vi "Meas Config Panel.vi"(8 "error in":errorcluster, 9 "force no GUI (False)":bool, 10 "always show setup (False)":bool, 11 "session in":T91={"adc"={"niScope"={"channel cfg"=[], "sessions"=[], "multi cards"=FALSE, "channels"=0, "type"=enum."n/a", "memory [B/chn]"=0, "ext. clock [Hz]"=0.0, "samples count"=0, "use streaming"=FALSE, "proc setup"={"packet size [smpl]"=0, "current timeout [s]"=0.0, "blk2blk timeout [s]"=0.0, "event time"=timestamp(0 s since 1904-01-01), "temp sampl T [s]"=0.0, "data queue"=refnum, "stop notifier"=refnum, "proc ref"=refnum}, "sample width [B]"=0, "ranges [V]"=[], "trigger setup"={"coupling"=1, "level [V]"=0.0, "slope"=0, "mode"=enum."Immediate", "pre-trigger [%]"=0.0}, "fs [Hz]"=0.0, "bitres [bit]"=0, "clock source"=enum."VAL_NO_SOURCE"}, "3458A"={"channels"=[], "sync unit"={"VISA"="", "type"=enum."Picotest U6200A"}, "awg unit"={"type"=enum."Agilent 331xxA to 332xxA", "VISA"="", "enable 10MHz ref"=FALSE, "cmi ckd2"={"VISA"="", "clock source"=enum."Auto", "manual ref clk"=FALSE, "ref clock [Hz]"=0.0, "div mode"=enum."Set divisor directly"}, "cmi sync v3"={"VISA"="", "baud rate [bd/s]"=115200, "source"=enum."Auto", "hv range"=enum."1kV", "fsrc is fixed"=FALSE, "fsrc [Hz]"=10000000.0, "freq integ [s]"=1.0, "freq filter"=5, "trig level"=enum."TTL 5V", "chn1 mode"=enum."Source divider", "chn1 level"=enum."Positive 5V", "chn2 mode"=enum."Source divider", "chn2 level"=enum."Positive 5V", "chn2 div"=1, "chn3 mode"=enum."Chn 1 Active", "chn3 level"=enum."Positive 5V", "chn1 div entry"=enum."Calculate nearest divisor from measured fx", "chn1 dev limit [%]"=1.0, "chn1 check dev"=FALSE}, "trigger"={"source"=enum."Immediate", "slope"=enum."POS", "coupling"=enum."DC", "level [V]"=0.0, "hysteresis [V]"=0.0, "pre-trigger [%]"=0.0}, "HMF2500 cfg"={"Baud Rate"=9600, "Parity"=0, "Data Bits"=8, "Flow Control"=4}}, "sync mode"=enum."MASTER-SLAVE, MASTER clocked by TIMER", "streaming mode"=FALSE, "idn mode"=enum."Auto", "sampling mode"=enum."DCV", "sample memory [B]"=0, "proc setup"={"channel id"=0, "packet size [smpl]"=0, "current timeout [s]"=0.0, "blk2blk timeout [s]"=0.0, "event time"=timestamp(0 s since 1904-01-01), "stop notifier"=refnum, "data queues"=[], "proc refs"=[], "bus semaphore"=refnum}, "sample size [B]"=0, "sample count"=0, "aux data"={"channel id"=0, "valid?"=[], "gain [V]"=[], "timestamp [s]"=[], "Ts [s]"=0.0, "abs timestamp"=timestamp(0 s since 1904-01-01), "t [deg C]"=[], "multiplex timestamp [s]"=-1.0, "only multiplex?"=FALSE, "multiplex smpl offset"=0, "overflow?"=FALSE}, "ranges [V]"=[], "aperture [s]"=0.0, "LEVEL trigger"={"edge"=enum."POS", "level [V]"=0.0, "coupling"=enum."DC"}, "trigger mode"=enum."AUTO", "measure temp.?"=FALSE, "disp mesages"=[], "shared bus?"=FALSE, "disable display?"=FALSE, "aper mode"=enum."Manual", "aper rules"=[], "multiplex"={"cycles"=0, "delay [s]"=0.0, "enabled"=FALSE, "overhead [s]"=1.0, "tot smpls"=0, "sub-rec"=0, "overhead [%]"=0.0, "emulated"=FALSE}, "F8588 lpf"=enum."Off", "F8588 pll"=enum."Off", "F8588 couple"=enum."DC, auto", "fs"={"freq mode"=enum."fs or Ts", "fs [Hz]"=0.0, "fref [Hz]"=0.0, "mul"=0.0, "div"=0.0}, "fs mode"=enum."fs or Ts", "init timestamp"=timestamp(0 s since 1904-01-01), "last report timestamp"=timestamp(0 s since 1904-01-01)}, "dsdll"={"dsdll"={"dsdll path"=path "", "dsdll handle"=[], "output devices"=[], "capture devices"=[]}, "channels"=0, "device id"=0, "channel idns"=[], "proc setup"={"packet size [smpl]"=0, "current timeout [s]"=0.0, "blk2blk timeout [s]"=0.0, "event time"=timestamp(0 s since 1904-01-01), "data queue"=refnum, "stop notifier"=refnum, "proc ref"=refnum}, "samples count"=0, "fs [Hz]"=0.0}, "type"=enum."niScope", "channel idn str"=[], "aux instr idn str"=[], "modified?"=FALSE, "simadc"={"channels"=[], "range [V]"=0.0, "Ts step [s]"=0.0, "time [s]"=0.0, "fs [Hz]"=0.0, "count"=0, "smpl offset"=0, "set count"=0, "bit res"=0}, "force rst?"=FALSE, "exit mode"=enum."Immediate reset", "exit dly"=0.0, "exit tmr"=timestamp(0 s since 1904-01-01), "busy?"=FALSE, "accessed?"=FALSE, "multiplex"={"Type"=enum."Dummy", "gen com ssn"={"visa"="", "primary"=enum."None", "secondary"=enum."None", "channels"=[]}, "delay before [s]"=0.0, "delay post [s]"=0.0, "sequence"=[], "enabled"=FALSE, "ref timestamp [s]"=0.0, "idn string"="", "dev niScope"="", "niScope idx"=0, "QPMX ssn"={"visa"="", "switch mode"=enum."Switched by TWM", "sequence"=[], "timing delays"=[], "polarity"=enum."Positive", "ss delay (s)"=2.0, "internal timer (s)"=1.0, "Last loaded sequence file"=path "", "startup delay (s)"=2.0}, "VISA mux ssn"={"VISA"="", "paths"=[], "idn command"="", "serial cfg"={"Baud rate"=9600, "Data bits"=8, "Parity"=0, "Stop bits"=10, "Flow control"=0, "End Mode Read"=enum."None", "End Mode Write"=enum."None", "Term character"=0, "Term enable"=FALSE}}}, "keysight dso"={"VISA"="", "channels"=[], "bw limit [Hz]"=0.0, "resolution"=enum."Basic", "trig noise reject"=enum."Normal", "N"=0, "trigger config"={"trigger source"=enum."Immediate", "trigger slope"=enum."Negative", "level [V]"=0.0, "hysteresis [V]"=0.001, "pre-trig [%]"=50}, "fs [Hz]"=0.0, "timeout stop"=timestamp(0 s since 1904-01-01), "waiting for opc"=FALSE, "fetch offset [smpl]"=0, "abs timestamp"=timestamp(0 s since 1904-01-01), "ranges [V]"=[], "decimation"=1.0, "ext ref"=FALSE, "emulate aperture"=FALSE, "model"=enum."DSO91304"}, "cdaq"={"mclk [Hz]"=12800000.0, "ADC task"="", "mclk reference"="", "fs [Hz]"=50000.0, "queue adc cmd"=refnum, "queue adc data"=refnum, "adc proc ref"=refnum, "channels"=[], "last channels"=[], "timeout"=timestamp(0 s since 1904-01-01), "N"=1000, "mclk mode"=enum."Free running", "ext mclk source"=""}, "ignore overload"=FALSE, "ADS127L21"={"VISA"="", "chn list"=[], "record size"=0, "phys. channels"=0, "adc fifo size"=0, "channels"=[], "ext refclk?"=FALSE, "fs [Hz]"=0.0, "ext refclk [Hz]"=0.0, "meas refclk [Hz]"=0.0, "EXTOUT mode"=enum."ADCCLK", "EXTOUT polarity"=enum."NORM", "EXTOUT divisor"=0}}, "sequence"=[], "sequence setup"={"group setups"=[], "rec count"=0, "range mode"=enum."Keep defaults", "fs mode"=enum."Frequency", "rng even"=0.0, "rng odd"=0.0, "folder"=path "", "name base"="", "meas id"=0, "settle [s]"=0.0, "comment"="", "avg count"=0, "fs-abs-fr fr"=0.0, "fs-abs-fr fs"=0.0, "fs-div fr"=0.0, "fs-div div"=0.0, "fs-mn fr"=0.0, "fs-mn mul"=0.0, "fs-mn div"=0.0, "fs-rat fr"=0.0, "fs-rat rat"=0.0}, "golpi"=refnum, "processing setup"={"mode"=enum."Raw", "call after avgs?"=FALSE, "calculate?"=FALSE, "raw mode"={"command"="", "result mode"=enum."Display console output (only Octave)", "res variable"=""}, "QWTB"={"QWTB path"=path "", "alg filter path"="", "alg ids"=[], "alg parameters"=[], "parsed parameters"=[], "selected alg id"="", "selected unc mode"=enum."None", "qwtb mcc"=100, "qwtb timeout"=90, "qwtb covg"=95.0, "qwtb ofs"=0, "qwtb lim data"=0, "multicore"={"jobs folder"=path "", "cores"=0, "max jobs"=0, "mode"=enum."Singlecore"}, "unc once?"=FALSE, "qwtb tstemp"=enum."Enabled (default)", "octave reset"=FALSE, "exec mode"=enum."Single-core"}}, "corrections"={"transducers"={"channels"=[], "last path"=path "", "root path"=path ""}, "digitizer"={"last path"=path "", "channel paths"=[], "channel idns"=[], "correction name"="", "channel names"=[], "folders to copy"=[], "channel valid"=[], "correction path"=path "", "correction rel path"="", "rel folders to copy"=[], "root path"=path ""}}, "assist cfg"={"P"=0, "Q"=0, "rel shift"=0.0, "ref freq"=0.0, "min fs"=0.0, "max fs tol"=0.0, "min int"=0.0, "max int"=0.0, "max err"=0.0, "max timeout"=0.0}} {"corrections"."transducers"."channels"."Phase index" min=1 step=1; "adc"."ADS127L21"."channels"."Channel" min=1 max=8 step=1; "adc"."ADS127L21"."channels"."Range [Vpk]" items=["±1.65V", "±2V"]; "adc"."cdaq"."last channels"."Channel id" min=0 step=1; "adc"."cdaq"."channels"."Channel id" min=0 step=1; "adc"."keysight dso"."decimation" min=1.0; "adc"."keysight dso"."bw limit [Hz]" format="%#_6p"; "adc"."keysight dso"."channels"."Offset [V]" format="%#_6p"; "adc"."keysight dso"."channels"."Range [Vpk]" min=0.0 format="%#_6p"; "adc"."keysight dso"."channels"."Channel" min=1; "adc"."multiplex"."VISA mux ssn"."serial cfg"."Flow control" items=["None", "XON/XOFF", "CTS/RTS", "XON/XOFF + CTS/RTS", "DTR/DSR", "XON/XOFF + DTR/DSR"]; "adc"."multiplex"."VISA mux ssn"."serial cfg"."Stop bits" items=["1 bit"=10, "1.5 bits"=15, "2 bits"=20]; "adc"."multiplex"."VISA mux ssn"."serial cfg"."Parity" items=["None", "Odd", "Even", "Mark", "Space"]; "adc"."multiplex"."VISA mux ssn"."serial cfg"."Data bits" items=["5 bits"=5, "6 bits"=6, "7 bits"=7, "8 bits"=8]; "adc"."multiplex"."VISA mux ssn"."serial cfg"."Baud rate" items=["150 Bd"=150, "300 Bd"=300, "600 Bd"=600, "1200 Bd"=1200, "2400 Bd"=2400, "4800 Bd"=4800, "9600 Bd"=9600, "19.2 kBd"=19200, "38.4 kBd"=38400, "57.6 kBd"=57600, "115.2 kBd"=115200]; "adc"."multiplex"."QPMX ssn"."startup delay (s)" min=0.0 step=1.0; "adc"."multiplex"."QPMX ssn"."internal timer (s)" min=0.0 step=1.0; "adc"."multiplex"."QPMX ssn"."ss delay (s)" min=0.0 step=1.0; "adc"."multiplex"."QPMX ssn"."timing delays" min=1 max=255 step=1; "adc"."3458A"."awg unit"."HMF2500 cfg"."Flow Control" items=["None", "XON/XOFF", "RTS/CTS", "XON/XOFF & RTS/CTS", "DTR/DSR", "XON/XOFF & DTR/DSR"]; "adc"."3458A"."awg unit"."HMF2500 cfg"."Data Bits" items=["7"=7, "8"=8]; "adc"."3458A"."awg unit"."HMF2500 cfg"."Parity" items=["None", "Odd", "Even", "Mark", "Space"]; "adc"."3458A"."awg unit"."HMF2500 cfg"."Baud Rate" items=["300"=300, "600"=600, "1200"=1200, "2400"=2400, "4800"=4800, "9600"=9600, "19200"=19200]; "adc"."3458A"."awg unit"."cmi sync v3"."chn2 div" min=1 max=100000000 step=1; "adc"."3458A"."awg unit"."cmi sync v3"."fsrc [Hz]" format="%_8p"; "adc"."3458A"."channels"."Range [Vpk]" min=0.0; "adc"."niScope"."trigger setup"."pre-trigger [%]" format="%.2f"; "adc"."niScope"."trigger setup"."level [V]" format="%.2f"; "adc"."niScope"."trigger setup"."coupling" items=["AC"=0, "DC"=1, "HF Reject"=3, "LF Reject"=4, "AC Plus HF Reject"=1001]; "adc"."niScope"."channel cfg"."Range [Vpk]" min=0.0; "adc"."niScope"."channel cfg"."Channel" min=0}) -> (0 "error out":errorcluster, 2 "canceled?":bool, 3 "session out":T91={"adc"={"niScope"={"channel cfg"=[], "sessions"=[], "multi cards"=FALSE, "channels"=0, "type"=enum."n/a", "memory [B/chn]"=0, "ext. clock [Hz]"=0.0, "samples count"=0, "use streaming"=FALSE, "proc setup"={"packet size [smpl]"=0, "current timeout [s]"=0.0, "blk2blk timeout [s]"=0.0, "event time"=timestamp(0 s since 1904-01-01), "temp sampl T [s]"=0.0, "data queue"=refnum, "stop notifier"=refnum, "proc ref"=refnum}, "sample width [B]"=0, "ranges [V]"=[], "trigger setup"={"coupling"=1, "level [V]"=0.0, "slope"=0, "mode"=enum."Immediate", "pre-trigger [%]"=0.0}, "fs [Hz]"=0.0, "bitres [bit]"=0, "clock source"=enum."VAL_NO_SOURCE"}, "3458A"={"channels"=[], "sync unit"={"VISA"="", "type"=enum."Picotest U6200A"}, "awg unit"={"type"=enum."Agilent 331xxA to 332xxA", "VISA"="", "enable 10MHz ref"=FALSE, "cmi ckd2"={"VISA"="", "clock source"=enum."Auto", "manual ref clk"=FALSE, "ref clock [Hz]"=0.0, "div mode"=enum."Set divisor directly"}, "cmi sync v3"={"VISA"="", "baud rate [bd/s]"=115200, "source"=enum."Auto", "hv range"=enum."1kV", "fsrc is fixed"=FALSE, "fsrc [Hz]"=10000000.0, "freq integ [s]"=1.0, "freq filter"=5, "trig level"=enum."TTL 5V", "chn1 mode"=enum."Source divider", "chn1 level"=enum."Positive 5V", "chn2 mode"=enum."Source divider", "chn2 level"=enum."Positive 5V", "chn2 div"=1, "chn3 mode"=enum."Chn 1 Active", "chn3 level"=enum."Positive 5V", "chn1 div entry"=enum."Calculate nearest divisor from measured fx", "chn1 dev limit [%]"=1.0, "chn1 check dev"=FALSE}, "trigger"={"source"=enum."Immediate", "slope"=enum."POS", "coupling"=enum."DC", "level [V]"=0.0, "hysteresis [V]"=0.0, "pre-trigger [%]"=0.0}, "HMF2500 cfg"={"Baud Rate"=9600, "Parity"=0, "Data Bits"=8, "Flow Control"=4}}, "sync mode"=enum."MASTER-SLAVE, MASTER clocked by TIMER", "streaming mode"=FALSE, "idn mode"=enum."Auto", "sampling mode"=enum."DCV", "sample memory [B]"=0, "proc setup"={"channel id"=0, "packet size [smpl]"=0, "current timeout [s]"=0.0, "blk2blk timeout [s]"=0.0, "event time"=timestamp(0 s since 1904-01-01), "stop notifier"=refnum, "data queues"=[], "proc refs"=[], "bus semaphore"=refnum}, "sample size [B]"=0, "sample count"=0, "aux data"={"channel id"=0, "valid?"=[], "gain [V]"=[], "timestamp [s]"=[], "Ts [s]"=0.0, "abs timestamp"=timestamp(0 s since 1904-01-01), "t [deg C]"=[], "multiplex timestamp [s]"=-1.0, "only multiplex?"=FALSE, "multiplex smpl offset"=0, "overflow?"=FALSE}, "ranges [V]"=[], "aperture [s]"=0.0, "LEVEL trigger"={"edge"=enum."POS", "level [V]"=0.0, "coupling"=enum."DC"}, "trigger mode"=enum."AUTO", "measure temp.?"=FALSE, "disp mesages"=[], "shared bus?"=FALSE, "disable display?"=FALSE, "aper mode"=enum."Manual", "aper rules"=[], "multiplex"={"cycles"=0, "delay [s]"=0.0, "enabled"=FALSE, "overhead [s]"=1.0, "tot smpls"=0, "sub-rec"=0, "overhead [%]"=0.0, "emulated"=FALSE}, "F8588 lpf"=enum."Off", "F8588 pll"=enum."Off", "F8588 couple"=enum."DC, auto", "fs"={"freq mode"=enum."fs or Ts", "fs [Hz]"=0.0, "fref [Hz]"=0.0, "mul"=0.0, "div"=0.0}, "fs mode"=enum."fs or Ts", "init timestamp"=timestamp(0 s since 1904-01-01), "last report timestamp"=timestamp(0 s since 1904-01-01)}, "dsdll"={"dsdll"={"dsdll path"=path "", "dsdll handle"=[], "output devices"=[], "capture devices"=[]}, "channels"=0, "device id"=0, "channel idns"=[], "proc setup"={"packet size [smpl]"=0, "current timeout [s]"=0.0, "blk2blk timeout [s]"=0.0, "event time"=timestamp(0 s since 1904-01-01), "data queue"=refnum, "stop notifier"=refnum, "proc ref"=refnum}, "samples count"=0, "fs [Hz]"=0.0}, "type"=enum."niScope", "channel idn str"=[], "aux instr idn str"=[], "modified?"=FALSE, "simadc"={"channels"=[], "range [V]"=0.0, "Ts step [s]"=0.0, "time [s]"=0.0, "fs [Hz]"=0.0, "count"=0, "smpl offset"=0, "set count"=0, "bit res"=0}, "force rst?"=FALSE, "exit mode"=enum."Immediate reset", "exit dly"=0.0, "exit tmr"=timestamp(0 s since 1904-01-01), "busy?"=FALSE, "accessed?"=FALSE, "multiplex"={"Type"=enum."Dummy", "gen com ssn"={"visa"="", "primary"=enum."None", "secondary"=enum."None", "channels"=[]}, "delay before [s]"=0.0, "delay post [s]"=0.0, "sequence"=[], "enabled"=FALSE, "ref timestamp [s]"=0.0, "idn string"="", "dev niScope"="", "niScope idx"=0, "QPMX ssn"={"visa"="", "switch mode"=enum."Switched by TWM", "sequence"=[], "timing delays"=[], "polarity"=enum."Positive", "ss delay (s)"=2.0, "internal timer (s)"=1.0, "Last loaded sequence file"=path "", "startup delay (s)"=2.0}, "VISA mux ssn"={"VISA"="", "paths"=[], "idn command"="", "serial cfg"={"Baud rate"=9600, "Data bits"=8, "Parity"=0, "Stop bits"=10, "Flow control"=0, "End Mode Read"=enum."None", "End Mode Write"=enum."None", "Term character"=0, "Term enable"=FALSE}}}, "keysight dso"={"VISA"="", "channels"=[], "bw limit [Hz]"=0.0, "resolution"=enum."Basic", "trig noise reject"=enum."Normal", "N"=0, "trigger config"={"trigger source"=enum."Immediate", "trigger slope"=enum."Negative", "level [V]"=0.0, "hysteresis [V]"=0.001, "pre-trig [%]"=50}, "fs [Hz]"=0.0, "timeout stop"=timestamp(0 s since 1904-01-01), "waiting for opc"=FALSE, "fetch offset [smpl]"=0, "abs timestamp"=timestamp(0 s since 1904-01-01), "ranges [V]"=[], "decimation"=1.0, "ext ref"=FALSE, "emulate aperture"=FALSE, "model"=enum."DSO91304"}, "cdaq"={"mclk [Hz]"=12800000.0, "ADC task"="", "mclk reference"="", "fs [Hz]"=50000.0, "queue adc cmd"=refnum, "queue adc data"=refnum, "adc proc ref"=refnum, "channels"=[], "last channels"=[], "timeout"=timestamp(0 s since 1904-01-01), "N"=1000, "mclk mode"=enum."Free running", "ext mclk source"=""}, "ignore overload"=FALSE, "ADS127L21"={"VISA"="", "chn list"=[], "record size"=0, "phys. channels"=0, "adc fifo size"=0, "channels"=[], "ext refclk?"=FALSE, "fs [Hz]"=0.0, "ext refclk [Hz]"=0.0, "meas refclk [Hz]"=0.0, "EXTOUT mode"=enum."ADCCLK", "EXTOUT polarity"=enum."NORM", "EXTOUT divisor"=0}}, "sequence"=[], "sequence setup"={"group setups"=[], "rec count"=0, "range mode"=enum."Keep defaults", "fs mode"=enum."Frequency", "rng even"=0.0, "rng odd"=0.0, "folder"=path "", "name base"="", "meas id"=0, "settle [s]"=0.0, "comment"="", "avg count"=0, "fs-abs-fr fr"=0.0, "fs-abs-fr fs"=0.0, "fs-div fr"=0.0, "fs-div div"=0.0, "fs-mn fr"=0.0, "fs-mn mul"=0.0, "fs-mn div"=0.0, "fs-rat fr"=0.0, "fs-rat rat"=0.0}, "golpi"=refnum, "processing setup"={"mode"=enum."Raw", "call after avgs?"=FALSE, "calculate?"=FALSE, "raw mode"={"command"="", "result mode"=enum."Display console output (only Octave)", "res variable"=""}, "QWTB"={"QWTB path"=path "", "alg filter path"="", "alg ids"=[], "alg parameters"=[], "parsed parameters"=[], "selected alg id"="", "selected unc mode"=enum."None", "qwtb mcc"=100, "qwtb timeout"=90, "qwtb covg"=95.0, "qwtb ofs"=0, "qwtb lim data"=0, "multicore"={"jobs folder"=path "", "cores"=0, "max jobs"=0, "mode"=enum."Singlecore"}, "unc once?"=FALSE, "qwtb tstemp"=enum."Enabled (default)", "octave reset"=FALSE, "exec mode"=enum."Single-core"}}, "corrections"={"transducers"={"channels"=[], "last path"=path "", "root path"=path ""}, "digitizer"={"last path"=path "", "channel paths"=[], "channel idns"=[], "correction name"="", "channel names"=[], "folders to copy"=[], "channel valid"=[], "correction path"=path "", "correction rel path"="", "rel folders to copy"=[], "root path"=path ""}}, "assist cfg"={"P"=0, "Q"=0, "rel shift"=0.0, "ref freq"=0.0, "min fs"=0.0, "max fs tol"=0.0, "min int"=0.0, "max int"=0.0, "max err"=0.0, "max timeout"=0.0}} {"corrections"."transducers"."channels"."Phase index" min=1 step=1; "adc"."ADS127L21"."channels"."Channel" min=1 max=8 step=1; "adc"."ADS127L21"."channels"."Range [Vpk]" items=["±1.65V", "±2V"]; "adc"."cdaq"."last channels"."Channel id" min=0 step=1; "adc"."cdaq"."channels"."Channel id" min=0 step=1; "adc"."keysight dso"."decimation" min=1.0; "adc"."keysight dso"."bw limit [Hz]" format="%#_6p"; "adc"."keysight dso"."channels"."Offset [V]" format="%#_6p"; "adc"."keysight dso"."channels"."Range [Vpk]" min=0.0 format="%#_6p"; "adc"."keysight dso"."channels"."Channel" min=1; "adc"."multiplex"."VISA mux ssn"."serial cfg"."Flow control" items=["None", "XON/XOFF", "CTS/RTS", "XON/XOFF + CTS/RTS", "DTR/DSR", "XON/XOFF + DTR/DSR"]; "adc"."multiplex"."VISA mux ssn"."serial cfg"."Stop bits" items=["1 bit"=10, "1.5 bits"=15, "2 bits"=20]; "adc"."multiplex"."VISA mux ssn"."serial cfg"."Parity" items=["None", "Odd", "Even", "Mark", "Space"]; "adc"."multiplex"."VISA mux ssn"."serial cfg"."Data bits" items=["5 bits"=5, "6 bits"=6, "7 bits"=7, "8 bits"=8]; "adc"."multiplex"."VISA mux ssn"."serial cfg"."Baud rate" items=["150 Bd"=150, "300 Bd"=300, "600 Bd"=600, "1200 Bd"=1200, "2400 Bd"=2400, "4800 Bd"=4800, "9600 Bd"=9600, "19.2 kBd"=19200, "38.4 kBd"=38400, "57.6 kBd"=57600, "115.2 kBd"=115200]; "adc"."multiplex"."QPMX ssn"."startup delay (s)" min=0.0 step=1.0; "adc"."multiplex"."QPMX ssn"."internal timer (s)" min=0.0 step=1.0; "adc"."multiplex"."QPMX ssn"."ss delay (s)" min=0.0 step=1.0; "adc"."multiplex"."QPMX ssn"."timing delays" min=1 max=255 step=1; "adc"."3458A"."awg unit"."HMF2500 cfg"."Flow Control" items=["None", "XON/XOFF", "RTS/CTS", "XON/XOFF & RTS/CTS", "DTR/DSR", "XON/XOFF & DTR/DSR"]; "adc"."3458A"."awg unit"."HMF2500 cfg"."Data Bits" items=["7"=7, "8"=8]; "adc"."3458A"."awg unit"."HMF2500 cfg"."Parity" items=["None", "Odd", "Even", "Mark", "Space"]; "adc"."3458A"."awg unit"."HMF2500 cfg"."Baud Rate" items=["300"=300, "600"=600, "1200"=1200, "2400"=2400, "4800"=4800, "9600"=9600, "19200"=19200]; "adc"."3458A"."awg unit"."cmi sync v3"."chn2 div" min=1 max=100000000 step=1; "adc"."3458A"."awg unit"."cmi sync v3"."fsrc [Hz]" format="%_8p"; "adc"."3458A"."channels"."Range [Vpk]" min=0.0; "adc"."niScope"."trigger setup"."pre-trigger [%]" format="%.2f"; "adc"."niScope"."trigger setup"."level [V]" format="%.2f"; "adc"."niScope"."trigger setup"."coupling" items=["AC"=0, "DC"=1, "HF Reject"=3, "LF Reject"=4, "AC Plus HF Reject"=1001]; "adc"."niScope"."channel cfg"."Range [Vpk]" min=0.0; "adc"."niScope"."channel cfg"."Channel" min=0})   [LabVIEW 2020]
doc: "New measurement configuration panel."
uses:
  Meas Session.ctl
  adc/ADC Session.ctl
  drivers/niScope/niScope Session.ctl
  drivers/niScope/niScope Virtual Channel Config.ctl
  drivers/niScope/niScope Virtual Channel Mode.ctl
  drivers/niScope/niScope Virtual Channel Input Z.ctl
  drivers/niScope/niScope Virtual Channel Coupling.ctl
  drivers/niScope/niScope Type.ctl
  drivers/niScope/niScope Digitizing Process Options.ctl
  drivers/niScope/niScope Data Packet.ctl
  drivers/niScope/niScope Trigger Setup.ctl
  <instrlib>/niScope/Controls/niScope trigger coupling.ctl
  <instrlib>/niScope/Controls/niScope trigger slope.ctl
  drivers/niScope/niScope Reference Clock.ctl
  drivers/DMM/3458A Digitizer Session.ctl
  drivers/DMM/3458A Virtual Channel Config.ctl
  drivers/Counter/Counter Session.ctl
  drivers/Counter/Counter Type.ctl
  drivers/AWG/AWG Session.ctl
  drivers/AWG/AWG Type.ctl
  drivers/AWG/CMI Clock Divider v2/CMI ckd2 Session.ctl
  drivers/AWG/CMI Clock Divider v2/CMI ckd2 Source Mode.ctl
  drivers/AWG/CMI Clock Divider v2/CMI ckd2 Divisor Mode.ctl
  drivers/AWG/CMI Sync V3/CMI Sync V3 session.ctl
  drivers/AWG/CMI Sync V3/Configure/CMI Sync V3 Reference Clock Source.ctl
  drivers/AWG/CMI Sync V3/Configure/CMI Sync V3 HV input Range.ctl
  drivers/AWG/CMI Sync V3/Configure/CMI Sync V3 Trigger Input Level.ctl
  drivers/AWG/CMI Sync V3/Configure/CMI Sync V3 Channel 1 Mode.ctl
  drivers/AWG/CMI Sync V3/Configure/CMI Sync V3 Channel Output Levels.ctl
  drivers/AWG/CMI Sync V3/Configure/CMI Sync V3 Channel 2 Mode.ctl
  drivers/AWG/CMI Sync V3/Configure/CMI Sync V3 Channel 3 Mode.ctl
  drivers/AWG/CMI Sync V3/Configure/CMI Sync V3 Channel 1 Divisor Entry Mode.ctl
  adc/ADC Trig Config.ctl
  adc/ADC Trig Mode Source.ctl
  adc/ADC Trig Slope.ctl
  adc/ADC Trig Coupling.ctl
  drivers/AWG/RaS HMF2500/HMF2500 Config.ctl
  drivers/DMM/3458A Sync Mode.ctl
  drivers/DMM/3458A Idn Mode.ctl
  drivers/DMM/3458A Digitizing Low Levels/Configure/Sampling Mode.ctl
  drivers/DMM/3458A Digitizing Process Options.ctl
  drivers/DMM/3458A Data Packet.ctl
  drivers/DMM/3458A Aux Record Data.ctl
  drivers/DMM/3458A Digitizing Low Levels/Configure/Level Setup.ctl
  drivers/DMM/3458A Digitizing Low Levels/Configure/First Sample Trigger.ctl
  drivers/DMM/3458A Aperture Selection Mode.ctl
  drivers/DMM/3458A Multiplexing Config.ctl
  drivers/Fluke 8588A/F8588A Low Pass Filter.ctl
  drivers/Fluke 8588A/F8588A Phase Lock.ctl
  drivers/Fluke 8588A/F8588A Coupling.ctl
  drivers/DMM/3458A Sampling Rate.ctl
  drivers/AWG/AWG Clock Setup Mode.ctl
  drivers/DMM/3458A Sample Rate Mode.ctl
  drivers/dsdll/DSDLL Session.ctl
  drivers/dsdll/dsdll/dsdll_instance.ctl
  drivers/dsdll/dsdll/dsdll_device_record.ctl
  drivers/dsdll/DSDLL Process Config.ctl
  drivers/dsdll/DSDLL Data Packet.ctl
  adc/ADC Type.ctl
  drivers/simulated_adc/SimAdc Config.ctl
  drivers/simulated_adc/SimAdc Channel Cfg.ctl
  adc/ADC On Close Action.ctl
  adc/Multiplexer/MPX Session.ctl
  adc/Multiplexer/MPX Type.ctl
  drivers/Multiplexers/Generic COM/GCOMM Session.ctl
  drivers/Multiplexers/Generic COM/GCOMM Signal.ctl
  drivers/Multiplexers/Generic COM/GCOMM Virtual Channel.ctl
  drivers/Multiplexers/Generic COM/GCOMM Logic State.ctl
  drivers/Multiplexers/Generic COM/QPMX Session.ctl
  drivers/Multiplexers/QPMX/QPMX switch mode.ctl
  drivers/Multiplexers/QPMX/QPMX polarity.ctl
  drivers/Multiplexers/Generic VISA commands/GVISA Mux Session.ctl
  drivers/Multiplexers/Generic VISA commands/GVISA Mux Path Entry.ctl
  drivers/Multiplexers/Generic VISA commands/met_serial_setup.ctl
  drivers/Agilent DSO 90000/Virtual Digitizer/KeDSO session.ctl
  drivers/Agilent DSO 90000/Virtual Digitizer/KeDSO Virtual Channel.ctl
  drivers/Agilent DSO 90000/Virtual Digitizer/KeDSO High Resolution Mode.ctl
  drivers/Agilent DSO 90000/Virtual Digitizer/KeDSO Trigger Setup.ctl
  drivers/Agilent DSO 90000/Virtual Digitizer/KeDSO Trigger Source.ctl
  drivers/Agilent DSO 90000/Public/Utility/DSO type.ctl
  drivers/cdaq/cDAQ Session.ctl
  drivers/cdaq/low_level_old/cdaq_anal_adc_command.ctl
  drivers/cdaq/low_level_old/cdaq_anal_adc_data.ctl
  drivers/cdaq/cDAQ Virtual Channel.ctl
  drivers/cdaq/cDAQ Master Clock Mode.ctl
  drivers/CMI_ADS127L21/CMI ADS127L21 - Session.ctl
  drivers/CMI_ADS127L21/CMI ADS127L21 - Record Channel.ctl
  drivers/CMI_ADS127L21/CMI ADS127L21 - Input Range.ctl
  drivers/CMI_ADS127L21/CMI ADS127L21 - Input Mode.ctl
  drivers/CMI_ADS127L21/CMI ADS127L21 - Input Impedance.ctl
  drivers/CMI_ADS127L21/CMI ADS127L21 - EXTOUT Mode.ctl
  drivers/CMI_ADS127L21/CMI ADS127L21 - EXTOUT Polarity.ctl
  Meas Sequence Item.ctl
  Meas Sampling Configuration.ctl
  processing/QWTB/Meas Proc QWTB Algorithm Parameter Data.ctl
  Meas Sequence Configuration.ctl
  Meas Range Mode.ctl
  Meas Sampling Rate Mode.ctl
  octave/golpi/mpc/golpi_session_ref.ctl
  octave/golpi/mpc/golpi_session.ctl
  octave/golpi/GOLPI reference Type Def.ctl
  octave/golpi/Pipe Handle.ctl
  processing/Meas Process Config.ctl
  processing/Meas Process Mode.ctl
  processing/Meas Process Raw Config.ctl
  processing/Meas Process Raw Result Mode.ctl
  processing/QWTB/Meas Proc QWTB Setup.ctl
  processing/QWTB/Meas Proc QWTB Uncertainty Mode.ctl
  processing/QWTB/Meas Proc QWTB Multicore Setup.ctl
  processing/QWTB/Meas Proc QWTB Multicore Type.ctl
  processing/Meas Process Time Stamp Mode.ctl
  processing/QWTB/Meas Proc QWTB Exec Mode.ctl
  Corrections/Corr Setup.ctl
  Corrections/Corr Tranducer Item.ctl
  Corrections/Corr Digitizers.ctl
  Assist/Assist Panel Setup.ctl
  varilib/SGUI Assign References Mode.ctl
  other/GUI Panel Control Action.ctl
  adc/ADC Capabilities Parameters.ctl
  varilib/SGUI Set Multiple Reals By Label.vi
  varilib/SGUI Set Single Real By Label.vi
  varilib/SGUI Set Single Integer By Label.vi
  varilib/varilib.lvlib
  drivers/AWG/AWG.lvlib
  drivers/DMM/3458A Virtual Digitizer.lvlib
  drivers/niScope/niScope Virtual Digitizer.lvlib
  drivers/Counter/Counter.lvlib
  drivers/DMM/3458A Digitizing Low Levels/3458A Digitizing Low Levels.lvlib
  drivers/dsdll/DSDLL Virtual Digitizer.lvlib
  octave/golpi/GOLPI library.lvlib
  octave/golpi/mpc/GOLPI Multi Process.lvlib
  drivers/dsdll/dsdll/dsdll.lvlib
  octave/golpi/LV Process library.lvlib
  drivers/AWG/CMI Sync V3/CMI Sync Unit V3.lvlib
  drivers/Agilent DSO 90000/Agilent 90000 Series.lvlib
panel:
  in  "pre-trig ratio":dbl=1e-06 caption="Pre-trigger ratio [%]" min=0.0 max=100.0 step=1.0 format="%#_3f"
  in  "trig hyst":dbl=1e-06 caption="Hysteresis [V]" min=1e-06 format="%#_3p"
  in  "btn default":bool
  in  "srate tabs":T1(tab)
  in  "fs mode":T2 caption="Sampling rate mode"
  in  "smpl rate":dbl caption="Sampling rate [Hz]" min=0.0 format="%_9p"
  out "smpl rate min":dbl caption="Sampling rate range [Hz]" format="%#_5p"
  out "smpl rate max":dbl caption="smpl rate min" format="%#_5p"
  out "smpl rate abs fr min":dbl caption="Sampling rate range [Hz]" format="%#_5p"
  out "smpl rate abs fr max":dbl caption="smpl rate min" format="%#_5p"
  in  "smpl abs fr fs":dbl caption="Sampling rate [Hz]" min=0.0 format="%_8p"
  in  "smpl abs fr":dbl caption="Reference frequency [Hz]" min=0.0 format="%_8p"
  out "smpl rate fr/N min":dbl caption="Sampling rate range [Hz]" format="%#_5p"
  out "smpl rate fr/N max":dbl caption="smpl rate min" format="%#_5p"
  out "smpl fr/N fs":dbl caption="Sampling rate [Hz]" min=0.0 format="%_8p"
  in  "smpl fr/N div":dbl=1.0 caption="Divisor" min=1.0 max=10000000.0 step=1.0
  in  "smpl fr/N fr":dbl caption="Reference frequency [Hz]" min=0.0 format="%_8p"
  in  "smpl fr*M/N mul":dbl=1.0 caption="Multiplier" min=1.0 max=10000000.0 step=1.0
  out "smpl rate fr*M/N min":dbl caption="Sampling rate range [Hz]" format="%#_5p"
  out "smpl rate fr*M/N max":dbl caption="smpl rate min" format="%#_5p"
  out "smpl fr*M/N fs":dbl caption="Sampling rate [Hz]" min=0.0 format="%_8p"
  in  "smpl fr*M/N div":dbl=1.0 caption="Divisor" min=1.0 max=10000000.0 step=1.0
  in  "smpl fr*M/N fr":dbl caption="Reference freq [Hz]" min=0.0 format="%_8p"
  in  "smpl fr*R fr":dbl caption="Reference frequency [Hz]" min=0.0 format="%_8p"
  in  "smpl fr*R rat":dbl=1.0 caption="Ratio" min=0.0 max=100000000.0 step=0.1 format="%_8g"
  out "smpl fr*R fs":dbl caption="Sampling rate [Hz]" min=0.0 format="%_8p"
  out "smpl rate fr*R max":dbl caption="smpl rate min" format="%#_5p"
  out "smpl rate fr*R min":dbl caption="Sampling rate range [Hz]" format="%#_5p"
  out "fs fixed":dbl caption="Sampling rate [Hz]" format="%_8p"
  out "fs info":string
  out "aper info":string
  in  "avg cycles":i32=1 caption="Sub-records count (averaging)" min=1
  in  "comment":string caption="Measurement comment"
  in  "rec delay":dbl caption="Pre-record settling [s]" min=0.0
  in  "btn assist":bool
  in  "smpl time":dbl caption="Meas. time [s]" min=0.0
  out "smpl time max":dbl caption="Max. time [s]" format="%#_6p"
  out "meas full":path caption="Full measurement base path preview"
  in  "meas id":i32 caption="Measurement number" min=0 max=9999 step=1
  in  "btn proc":bool
  in  "calc result?":bool caption="Enable result calculation?"
  in  "meas name":string caption="Measurement name base"
  in  "data folder":path caption="Folder for measurements data files"
  in  "rec cycles":i32=1 caption="Records count" min=1
  in  "range even":dbl
  in  "range odd":dbl
  in  "range mode":T3 caption="Voltage range selection"
  out "smpl count max":dbl caption="Max. samples count" format="%#_6p"
  in  "smpl count":i64=1 caption="Samples count" min=1
  out "aperture max":dbl caption="smpl rate min" format="%#_5p"
  out "aperture min":dbl caption="Aperture range [s]" format="%#_5p"
  in  "trig coupling":T4 caption="Trigger coupling"
  in  "trig slope":T5 caption="Trigger slope"
  in  "trig level":dbl caption="Level [V]" format="%#_3p"
  in  "trig mode":T6 caption="Trigger mode"
  in  "aperture":dbl caption="Aperture [s]" format="%#_3p"
  out "adc":T7={"niScope"={"channel cfg"=[], "sessions"=[], "multi cards"=FALSE, "channels"=0, "type"=enum."n/a", "memory [B/chn]"=0, "ext. clock [Hz]"=0.0, "samples count"=0, "use streaming"=FALSE, "proc setup"={"packet size [smpl]"=0, "current timeout [s]"=0.0, "blk2blk timeout [s]"=0.0, "event time"=timestamp(0 s since 1904-01-01), "temp sampl T [s]"=0.0, "data queue"=refnum, "stop notifier"=refnum, "proc ref"=refnum}, "sample width [B]"=0, "ranges [V]"=[], "trigger setup"={"coupling"=1, "level [V]"=0.0, "slope"=0, "mode"=enum."Immediate", "pre-trigger [%]"=0.0}, "fs [Hz]"=0.0, "bitres [bit]"=0, "clock source"=enum."VAL_NO_SOURCE"}, "3458A"={"channels"=[], "sync unit"={"VISA"="", "type"=enum."Picotest U6200A"}, "awg unit"={"type"=enum."Agilent 331xxA to 332xxA", "VISA"="", "enable 10MHz ref"=FALSE, "cmi ckd2"={"VISA"="", "clock source"=enum."Auto", "manual ref clk"=FALSE, "ref clock [Hz]"=0.0, "div mode"=enum."Set divisor directly"}, "cmi sync v3"={"VISA"="", "baud rate [bd/s]"=115200, "source"=enum."Auto", "hv range"=enum."1kV", "fsrc is fixed"=FALSE, "fsrc [Hz]"=10000000.0, "freq integ [s]"=1.0, "freq filter"=5, "trig level"=enum."TTL 5V", "chn1 mode"=enum."Source divider", "chn1 level"=enum."Positive 5V", "chn2 mode"=enum."Source divider", "chn2 level"=enum."Positive 5V", "chn2 div"=1, "chn3 mode"=enum."Chn 1 Active", "chn3 level"=enum."Positive 5V", "chn1 div entry"=enum."Calculate nearest divisor from measured fx", "chn1 dev limit [%]"=1.0, "chn1 check dev"=FALSE}, "trigger"={"source"=enum."Immediate", "slope"=enum."POS", "coupling"=enum."DC", "level [V]"=0.0, "hysteresis [V]"=0.0, "pre-trigger [%]"=0.0}, "HMF2500 cfg"={"Baud Rate"=9600, "Parity"=0, "Data Bits"=8, "Flow Control"=4}}, "sync mode"=enum."MASTER-SLAVE, MASTER clocked by TIMER", "streaming mode"=FALSE, "idn mode"=enum."Auto", "sampling mode"=enum."DCV", "sample memory [B]"=0, "proc setup"={"channel id"=0, "packet size [smpl]"=0, "current timeout [s]"=0.0, "blk2blk timeout [s]"=0.0, "event time"=timestamp(0 s since 1904-01-01), "stop notifier"=refnum, "data queues"=[], "proc refs"=[], "bus semaphore"=refnum}, "sample size [B]"=0, "sample count"=0, "aux data"={"channel id"=0, "valid?"=[], "gain [V]"=[], "timestamp [s]"=[], "Ts [s]"=0.0, "abs timestamp"=timestamp(0 s since 1904-01-01), "t [deg C]"=[], "multiplex timestamp [s]"=-1.0, "only multiplex?"=FALSE, "multiplex smpl offset"=0, "overflow?"=FALSE}, "ranges [V]"=[], "aperture [s]"=0.0, "LEVEL trigger"={"edge"=enum."POS", "level [V]"=0.0, "coupling"=enum."DC"}, "trigger mode"=enum."AUTO", "measure temp.?"=FALSE, "disp mesages"=[], "shared bus?"=FALSE, "disable display?"=FALSE, "aper mode"=enum."Manual", "aper rules"=[], "multiplex"={"cycles"=0, "delay [s]"=0.0, "enabled"=FALSE, "overhead [s]"=1.0, "tot smpls"=0, "sub-rec"=0, "overhead [%]"=0.0, "emulated"=FALSE}, "F8588 lpf"=enum."Off", "F8588 pll"=enum."Off", "F8588 couple"=enum."DC, auto", "fs"={"freq mode"=enum."fs or Ts", "fs [Hz]"=0.0, "fref [Hz]"=0.0, "mul"=0.0, "div"=0.0}, "fs mode"=enum."fs or Ts", "init timestamp"=timestamp(0 s since 1904-01-01), "last report timestamp"=timestamp(0 s since 1904-01-01)}, "dsdll"={"dsdll"={"dsdll path"=path "", "dsdll handle"=[], "output devices"=[], "capture devices"=[]}, "channels"=0, "device id"=0, "channel idns"=[], "proc setup"={"packet size [smpl]"=0, "current timeout [s]"=0.0, "blk2blk timeout [s]"=0.0, "event time"=timestamp(0 s since 1904-01-01), "data queue"=refnum, "stop notifier"=refnum, "proc ref"=refnum}, "samples count"=0, "fs [Hz]"=0.0}, "type"=enum."niScope", "channel idn str"=[], "aux instr idn str"=[], "modified?"=FALSE, "simadc"={"channels"=[], "range [V]"=0.0, "Ts step [s]"=0.0, "time [s]"=0.0, "fs [Hz]"=0.0, "count"=0, "smpl offset"=0, "set count"=0, "bit res"=0}, "force rst?"=FALSE, "exit mode"=enum."Immediate reset", "exit dly"=0.0, "exit tmr"=timestamp(0 s since 1904-01-01), "busy?"=FALSE, "accessed?"=FALSE, "multiplex"={"Type"=enum."Dummy", "gen com ssn"={"visa"="", "primary"=enum."None", "secondary"=enum."None", "channels"=[]}, "delay before [s]"=0.0, "delay post [s]"=0.0, "sequence"=[], "enabled"=FALSE, "ref timestamp [s]"=0.0, "idn string"="", "dev niScope"="", "niScope idx"=0, "QPMX ssn"={"visa"="", "switch mode"=enum."Switched by TWM", "sequence"=[], "timing delays"=[], "polarity"=enum."Positive", "ss delay (s)"=2.0, "internal timer (s)"=1.0, "Last loaded sequence file"=path "", "startup delay (s)"=2.0}, "VISA mux ssn"={"VISA"="", "paths"=[], "idn command"="", "serial cfg"={"Baud rate"=9600, "Data bits"=8, "Parity"=0, "Stop bits"=10, "Flow control"=0, "End Mode Read"=enum."None", "End Mode Write"=enum."None", "Term character"=0, "Term enable"=FALSE}}}, "keysight dso"={"VISA"="", "channels"=[], "bw limit [Hz]"=0.0, "resolution"=enum."Basic", "trig noise reject"=enum."Normal", "N"=0, "trigger config"={"trigger source"=enum."Immediate", "trigger slope"=enum."Negative", "level [V]"=0.0, "hysteresis [V]"=0.001, "pre-trig [%]"=50}, "fs [Hz]"=0.0, "timeout stop"=timestamp(0 s since 1904-01-01), "waiting for opc"=FALSE, "fetch offset [smpl]"=0, "abs timestamp"=timestamp(0 s since 1904-01-01), "ranges [V]"=[], "decimation"=1.0, "ext ref"=FALSE, "emulate aperture"=FALSE, "model"=enum."DSO91304"}, "cdaq"={"mclk [Hz]"=12800000.0, "ADC task"="", "mclk reference"="", "fs [Hz]"=50000.0, "queue adc cmd"=refnum, "queue adc data"=refnum, "adc proc ref"=refnum, "channels"=[], "last channels"=[], "timeout"=timestamp(0 s since 1904-01-01), "N"=1000, "mclk mode"=enum."Free running", "ext mclk source"=""}, "ignore overload"=FALSE, "ADS127L21"={"VISA"="", "chn list"=[], "record size"=0, "phys. channels"=0, "adc fifo size"=0, "channels"=[], "ext refclk?"=FALSE, "fs [Hz]"=0.0, "ext refclk [Hz]"=0.0, "meas refclk [Hz]"=0.0, "EXTOUT mode"=enum."ADCCLK", "EXTOUT polarity"=enum."NORM", "EXTOUT divisor"=0}} {"ADS127L21"."channels"."Channel" min=1 max=8 step=1; "ADS127L21"."channels"."Range [Vpk]" items=["±1.65V", "±2V"]; "cdaq"."last channels"."Channel id" min=0 step=1; "cdaq"."channels"."Channel id" min=0 step=1; "keysight dso"."decimation" min=1.0; "keysight dso"."bw limit [Hz]" format="%#_6p"; "keysight dso"."channels"."Offset [V]" format="%#_6p"; "keysight dso"."channels"."Range [Vpk]" min=0.0 format="%#_6p"; "keysight dso"."channels"."Channel" min=1; "multiplex"."VISA mux ssn"."serial cfg"."Flow control" items=["None", "XON/XOFF", "CTS/RTS", "XON/XOFF + CTS/RTS", "DTR/DSR", "XON/XOFF + DTR/DSR"]; "multiplex"."VISA mux ssn"."serial cfg"."Stop bits" items=["1 bit"=10, "1.5 bits"=15, "2 bits"=20]; "multiplex"."VISA mux ssn"."serial cfg"."Parity" items=["None", "Odd", "Even", "Mark", "Space"]; "multiplex"."VISA mux ssn"."serial cfg"."Data bits" items=["5 bits"=5, "6 bits"=6, "7 bits"=7, "8 bits"=8]; "multiplex"."VISA mux ssn"."serial cfg"."Baud rate" items=["150 Bd"=150, "300 Bd"=300, "600 Bd"=600, "1200 Bd"=1200, "2400 Bd"=2400, "4800 Bd"=4800, "9600 Bd"=9600, "19.2 kBd"=19200, "38.4 kBd"=38400, "57.6 kBd"=57600, "115.2 kBd"=115200]; "multiplex"."QPMX ssn"."startup delay (s)" min=0.0 step=1.0; "multiplex"."QPMX ssn"."internal timer (s)" min=0.0 step=1.0; "multiplex"."QPMX ssn"."ss delay (s)" min=0.0 step=1.0; "multiplex"."QPMX ssn"."timing delays" min=1 max=255 step=1; "3458A"."awg unit"."HMF2500 cfg"."Flow Control" items=["None", "XON/XOFF", "RTS/CTS", "XON/XOFF & RTS/CTS", "DTR/DSR", "XON/XOFF & DTR/DSR"]; "3458A"."awg unit"."HMF2500 cfg"."Data Bits" items=["7"=7, "8"=8]; "3458A"."awg unit"."HMF2500 cfg"."Parity" items=["None", "Odd", "Even", "Mark", "Space"]; "3458A"."awg unit"."HMF2500 cfg"."Baud Rate" items=["300"=300, "600"=600, "1200"=1200, "2400"=2400, "4800"=4800, "9600"=9600, "19200"=19200]; "3458A"."awg unit"."cmi sync v3"."chn2 div" min=1 max=100000000 step=1; "3458A"."awg unit"."cmi sync v3"."fsrc [Hz]" format="%_8p"; "3458A"."channels"."Range [Vpk]" min=0.0; "niScope"."trigger setup"."pre-trigger [%]" format="%.2f"; "niScope"."trigger setup"."level [V]" format="%.2f"; "niScope"."trigger setup"."coupling" items=["AC"=0, "DC"=1, "HF Reject"=3, "LF Reject"=4, "AC Plus HF Reject"=1001]; "niScope"."channel cfg"."Range [Vpk]" min=0.0; "niScope"."channel cfg"."Channel" min=0}
  in  "btn cancel":bool
  in  "btn ok":bool
  # "Use following variables in the name base:\n  %id% - measurement number in format DDDD\n  %date% - date of the measurement YYYYMMDD\n  %time% - time of the measurement HH-MM-SS\nExample:\n  my_measurement_%id%"
  # "ADC:"
  # "ADC:"
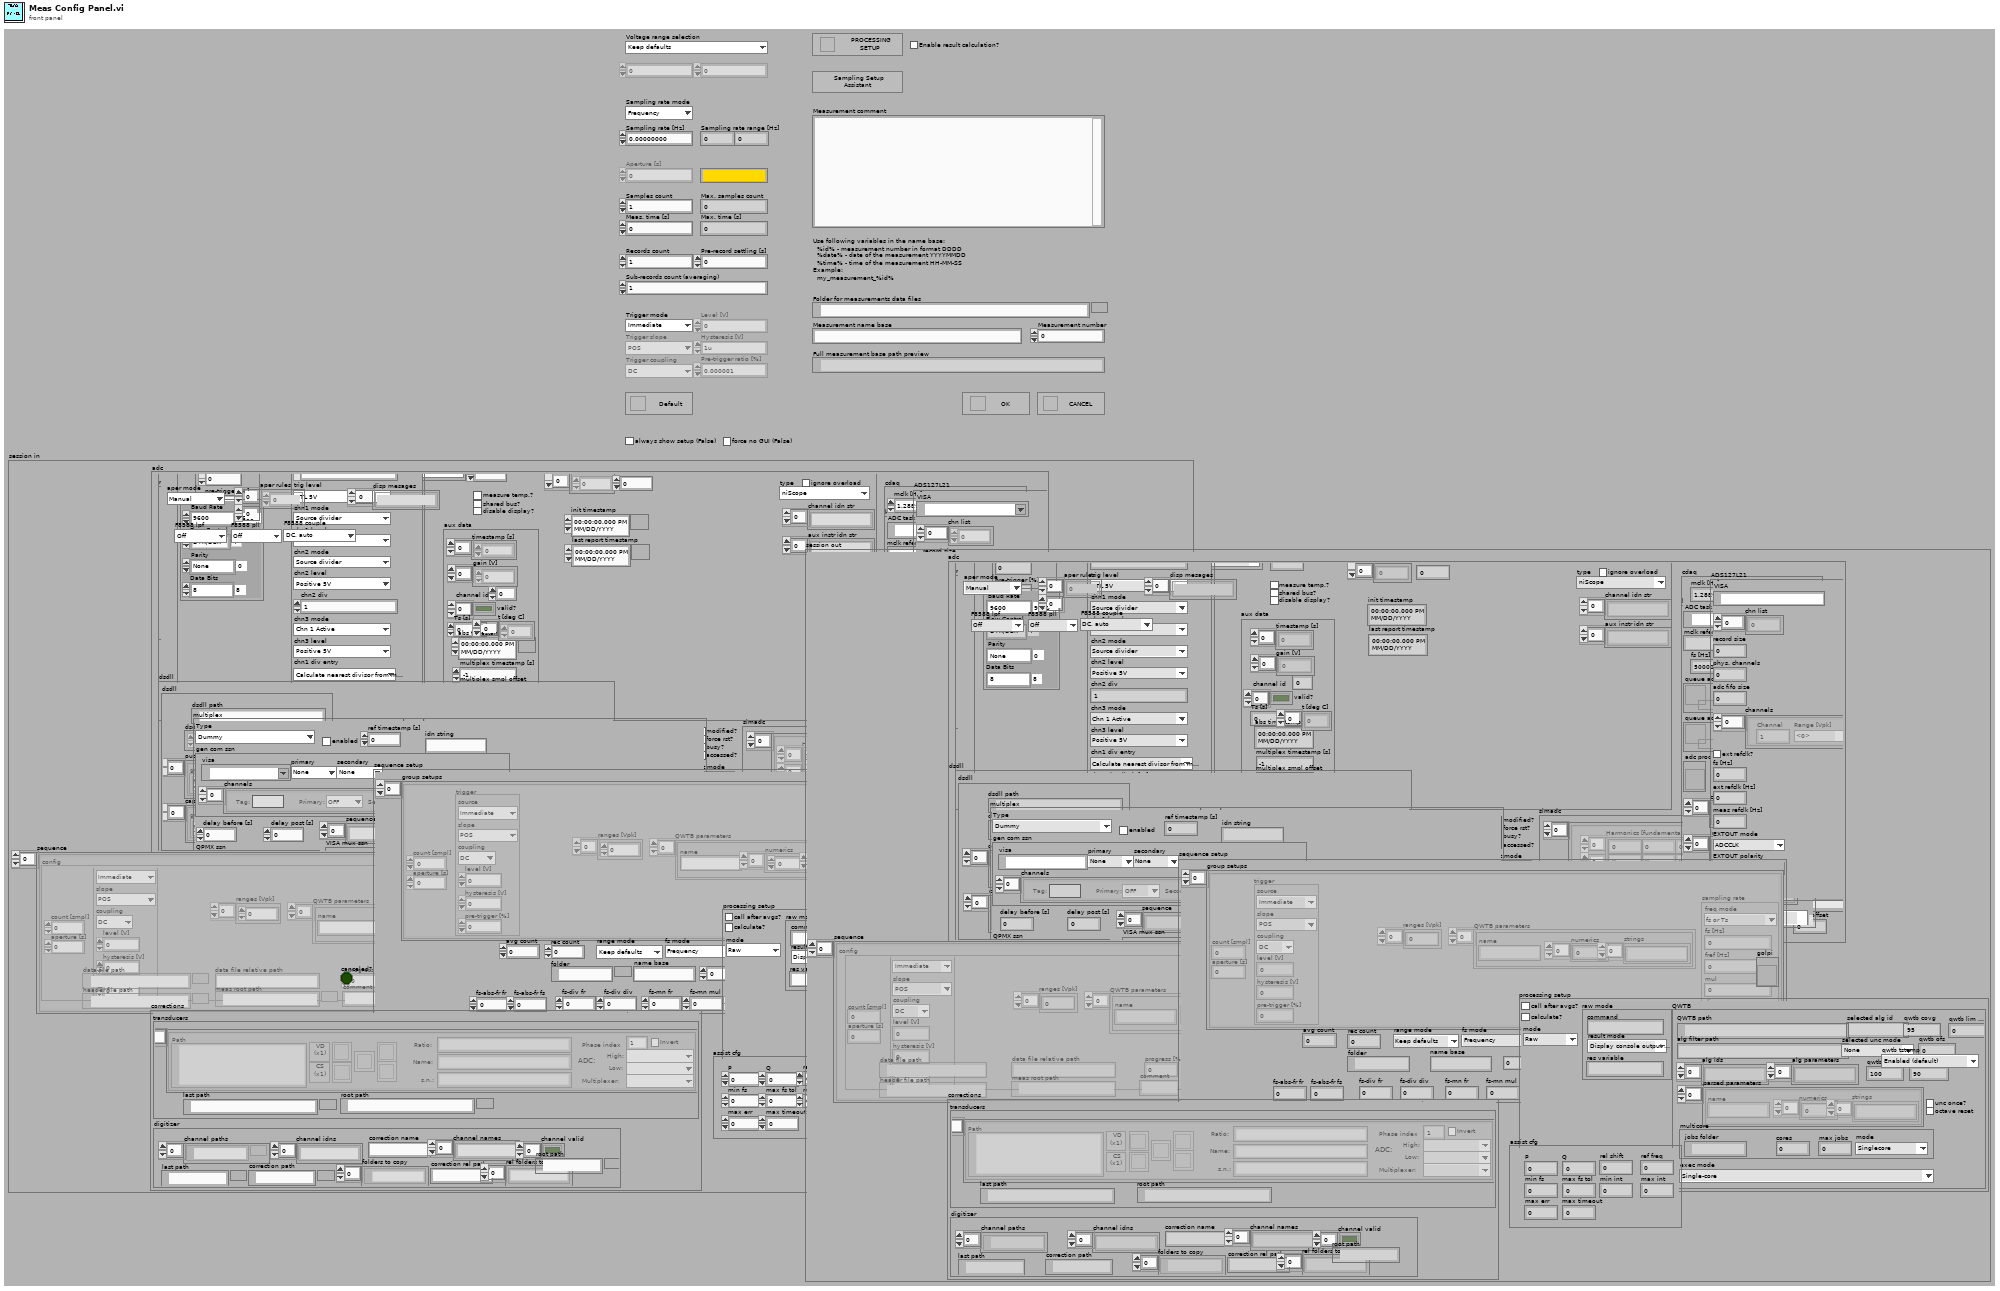
[diagram p1: front panel]
types:
  T1 = enum32{"abs", "abs fr", "fr/N", "fr*M/N", "fr*R", "fix"}
  T2 = typedef "Meas Sampling Rate Mode.ctl" = enum16{"Frequency", "Period"}
  T3 = typedef "Meas Range Mode.ctl" = enum16{"Keep defaults", "Set All channels", "Set Odd and Even channels"}
  T4 = typedef "ADC Trig Coupling.ctl" = enum16{"DC", "AC"}
  T5 = typedef "ADC Trig Slope.ctl" = enum16{"POS", "NEG"}
  T6 = typedef "ADC Trig Mode Source.ctl" = enum16{"Immediate", "External", "Level"}
  T7 = typedef "ADC Session.ctl" = cluster{"niScope":T8, "3458A":T19, "dsdll":T55, "type":T59, "channel idn str":string[], "aux instr idn str":string[], "modified?":bool, "simadc":T60, "force rst?":bool, "exit mode":T62, "exit dly":dbl, "exit tmr":timestamp, "busy?":bool, "accessed?":bool, "multiplex":T63, "keysight dso":T75, "cdaq":T81, "ignore overload":bool, "ADS127L21":T84}
  T8 = typedef "niScope Virtual Digitizer.lvlib/niScope Session.ctl" = cluster{"channel cfg":T9[], "sessions":refnum<k20>[], "multi cards":bool, "channels":i32, "type":T13, "memory [B/chn]":i32, "ext. clock [Hz]":dbl, "samples count":i64, "use streaming":bool, "proc setup":T14, "sample width [B]":i32, "ranges [V]":dbl[], "trigger setup":T15, "fs [Hz]":dbl, "bitres [bit]":i32, "clock source":T18}
  T9 = typedef "niScope Virtual Digitizer.lvlib/niScope Virtual Channel Config.ctl" = cluster{"Address":refnum<k15>, "Channel":i32, "Mode":T10, "Input Z":T11, "Coupling":T12, "Range [Vpk]":dbl, "btn clr":bool, "btn up":bool, "btn down":bool}
  T10 = typedef "niScope Virtual Digitizer.lvlib/niScope Virtual Channel Mode.ctl" = enum16{"Single ended", "Unbal. differential", "Differential"}
  T11 = typedef "niScope Virtual Digitizer.lvlib/niScope Virtual Channel Input Z.ctl" = enum16{"1 MOhm", "50 Ohm"}
  T12 = typedef "niScope Virtual Digitizer.lvlib/niScope Virtual Channel Coupling.ctl" = enum16{"AC", "DC", "GND"}
  T13 = typedef "niScope Virtual Digitizer.lvlib/niScope Type.ctl" = enum16{"n/a", "5922"}
  T14 = typedef "niScope Virtual Digitizer.lvlib/niScope Digitizing Process Options.ctl" = cluster{"packet size [smpl]":i64, "current timeout [s]":dbl, "blk2blk timeout [s]":dbl, "event time":timestamp, "temp sampl T [s]":dbl, "data queue":refnum<queue>, "stop notifier":refnum<notifier>, "proc ref":refnum<vi>}
  T15 = typedef "niScope Virtual Digitizer.lvlib/niScope Trigger Setup.ctl" = cluster{"coupling":T16, "level [V]":dbl, "slope":T17, "mode":enum16{"Immediate", "External", "Level"}, "pre-trigger [%]":dbl}
  T16 = typedef "niScope trigger coupling.ctl" = u16
  T17 = typedef "niScope trigger slope.ctl" = i32
  T18 = typedef "niScope Virtual Digitizer.lvlib/niScope Reference Clock.ctl" = enum16{"VAL_NO_SOURCE", "VAL_CLK_IN", "VAL_PXI_CLOCK", "VAL_EXTERNAL"}
  T19 = typedef "3458A Virtual Digitizer.lvlib/3458A Digitizer Session.ctl" = cluster{"channels":T20[], "sync unit":T21, "awg unit":T23, "sync mode":T39, "streaming mode":bool, "idn mode":T40, "sampling mode":T41, "sample memory [B]":i32, "proc setup":T42, "sample size [B]":i32, "sample count":i32, "aux data":T44, "ranges [V]":dbl[], "aperture [s]":dbl, "LEVEL trigger":T45, "trigger mode":T46, "measure temp.?":bool, "disp mesages":string[], "shared bus?":bool, "disable display?":bool, "aper mode":T47, "aper rules":dbl[][], "multiplex":T48, "F8588 lpf":T49, "F8588 pll":T50, "F8588 couple":T51, "fs":T52, "fs mode":T54, "init timestamp":timestamp, "last report timestamp":timestamp}
  T20 = typedef "3458A Virtual Digitizer.lvlib/3458A Virtual Channel Config.ctl" = cluster{"VISA":refnum<visa-resource-name>, "Range [Vpk]":dbl, "btn clr":bool, "btn up":bool, "btn down":bool, "F8588":bool, "F8588 guard":bool}
  T21 = typedef "Counter.lvlib/Counter Session.ctl" = cluster{"VISA":refnum<visa-resource-name>, "type":T22}
  T22 = typedef "Counter.lvlib/Counter Type.ctl" = enum16{"Picotest U6200A", "dummy"}
  T23 = typedef "AWG.lvlib/AWG Session.ctl" = cluster{"type":T24, "VISA":refnum<visa-resource-name>, "enable 10MHz ref":bool, "cmi ckd2":T25, "cmi sync v3":T28, "trigger":T37, "HMF2500 cfg":T38}
  T24 = typedef "AWG.lvlib/AWG Type.ctl" = enum16{"Agilent 331xxA to 332xxA", "Agilent 335xxA to 336xxA", "Tektronix AFG3101C", "R&S HMF25xx", "CMI Clock Divider v2", "CMI Sync Unit V3", "dummy"}
  T25 = typedef "AWG.lvlib/CMI ckd2 Session.ctl" = cluster{"VISA":refnum<visa-resource-name>, "clock source":T26, "manual ref clk":bool, "ref clock [Hz]":dbl, "div mode":T27}
  T26 = typedef "AWG.lvlib/CMI ckd2 Source Mode.ctl" = enum16{"Auto", "LF clock", "HF clock", "Internal"}
  T27 = typedef "AWG.lvlib/CMI ckd2 Divisor Mode.ctl" = enum16{"Set divisor directly", "Set divisor by frequency"}
  T28 = typedef "AWG.lvlib/CMI Sync Unit V3.lvlib/CMI Sync V3 session.ctl" = cluster{"VISA":refnum<visa-resource-name>, "baud rate [bd/s]":i32, "source":T29, "hv range":T30, "fsrc is fixed":bool, "fsrc [Hz]":dbl, "freq integ [s]":dbl, "freq filter":i32, "trig level":T31, "chn1 mode":T32, "chn1 level":T33, "chn2 mode":T34, "chn2 level":T33, "chn2 div":i32, "chn3 mode":T35, "chn3 level":T33, "chn1 div entry":T36, "chn1 dev limit [%]":dbl, "chn1 check dev":bool}
  T29 = typedef "AWG.lvlib/CMI Sync Unit V3.lvlib/CMI Sync V3 Reference Clock Source.ctl" = enum16{"Auto", "Internal", "Logic", "Sine", "HV"}
  T30 = typedef "AWG.lvlib/CMI Sync Unit V3.lvlib/CMI Sync V3 HV input Range.ctl" = enum16{"10V", "60V", "250V", "1kV"}
  T31 = typedef "AWG.lvlib/CMI Sync Unit V3.lvlib/CMI Sync V3 Trigger Input Level.ctl" = enum16{"LVCMOS 3V3", "TTL 5V"}
  T32 = typedef "AWG.lvlib/CMI Sync Unit V3.lvlib/CMI Sync V3 Channel 1 Mode.ctl" = enum16{"Source divider", "DDS absolute", "DDS ratio", "DDS ratio M/N"}
  T33 = typedef "AWG.lvlib/CMI Sync Unit V3.lvlib/CMI Sync V3 Channel Output Levels.ctl" = enum16{"Positive 3V3", "Negative 3V3", "Positive 5V", "Negative 5V"}
  T34 = typedef "AWG.lvlib/CMI Sync Unit V3.lvlib/CMI Sync V3 Channel 2 Mode.ctl" = enum16{"Source divider", "Chn 1 divide"}
  T35 = typedef "AWG.lvlib/CMI Sync Unit V3.lvlib/CMI Sync V3 Channel 3 Mode.ctl" = enum16{"Chn 1 Active", "Chn 2 Active", "Chn 1 Trigger", "Chn 2 Trigger", "Gate", "PPS", "10MHz"}
  T36 = typedef "AWG.lvlib/CMI Sync Unit V3.lvlib/CMI Sync V3 Channel 1 Divisor Entry Mode.ctl" = enum16{"Set divisor directly", "Calculate nearest divisor from measured fx"}
  T37 = typedef "ADC Trig Config.ctl" = cluster{"source":T6, "slope":T5, "coupling":T4, "level [V]":dbl, "hysteresis [V]":dbl, "pre-trigger [%]":dbl}
  T38 = typedef "AWG.lvlib/HMF2500 Config.ctl" = cluster{"Baud Rate":u32, "Parity":u16, "Data Bits":u16, "Flow Control":u16}
  T39 = typedef "3458A Virtual Digitizer.lvlib/3458A Sync Mode.ctl" = enum16{"MASTER-SLAVE, MASTER clocked by TIMER", "MASTER-SLAVE, MASTER clocked by AWG", "ALL clocked by AWG", "MASTER-SLAVE, ALL clocked by TIMER", "ALL clocked by AWG with DFLL"}
  T40 = typedef "3458A Virtual Digitizer.lvlib/3458A Idn Mode.ctl" = enum16{"Auto", "Sequential (chn A, chn B, ...)", "From calibration string"}
  T41 = typedef "3458A Virtual Digitizer.lvlib/3458A Digitizing Low Levels.lvlib/Sampling Mode.ctl" = enum16{"DCV", "DSDC", "DSAC"}
  T42 = typedef "3458A Virtual Digitizer.lvlib/3458A Digitizing Process Options.ctl" = cluster{"channel id":i32, "packet size [smpl]":i32, "current timeout [s]":dbl, "blk2blk timeout [s]":dbl, "event time":timestamp, "stop notifier":refnum<notifier>, "data queues":refnum<queue>[], "proc refs":refnum<vi>[], "bus semaphore":T43}
  T43 = typedef "Semaphore RefNum" = refnum<k1>
  T44 = typedef "3458A Virtual Digitizer.lvlib/3458A Aux Record Data.ctl" = cluster{"channel id":i32, "valid?":bool[], "gain [V]":dbl[], "timestamp [s]":dbl[], "Ts [s]":dbl, "abs timestamp":timestamp, "t [deg C]":dbl[], "multiplex timestamp [s]":dbl, "only multiplex?":bool, "multiplex smpl offset":i64, "overflow?":bool}
  T45 = typedef "3458A Virtual Digitizer.lvlib/3458A Digitizing Low Levels.lvlib/Level Setup.ctl" = cluster{"edge":enum16{"POS", "NEG"}, "level [V]":dbl, "coupling":enum16{"DC", "AC"}}
  T46 = typedef "3458A Virtual Digitizer.lvlib/3458A Digitizing Low Levels.lvlib/First Sample Trigger.ctl" = enum16{"AUTO", "EXT", "SYN", "SGL", "HOLD", "LEVEL"}
  T47 = typedef "3458A Virtual Digitizer.lvlib/3458A Aperture Selection Mode.ctl" = enum16{"Manual", "Maximum", "Table"}
  T48 = typedef "3458A Virtual Digitizer.lvlib/3458A Multiplexing Config.ctl" = cluster{"cycles":i32, "delay [s]":dbl, "enabled":bool, "overhead [s]":dbl, "tot smpls":i64, "sub-rec":i32, "overhead [%]":dbl, "emulated":bool}
  T49 = typedef "F8588A Low Pass Filter.ctl" = enum16{"Off", "100 kHz", "3 MHz"}
  T50 = typedef "F8588A Phase Lock.ctl" = enum16{"Off", "1 MHz", "10 MHz"}
  T51 = typedef "F8588A Coupling.ctl" = enum16{"AC, 1 MOhm", "AC, 10 MOhm", "DC, 1 MOhm", "DC, 10 MOhm", "DC, auto"}
  T52 = typedef "3458A Virtual Digitizer.lvlib/3458A Sampling Rate.ctl" = cluster{"freq mode":T53, "fs [Hz]":dbl, "fref [Hz]":dbl, "mul":dbl, "div":dbl}
  T53 = typedef "AWG.lvlib/AWG Clock Setup Mode.ctl" = enum16{"fs or Ts", "fs or Ts with fref", "fref/N", "fref*M/N", "fref*Ratio"}
  T54 = typedef "3458A Sample Rate Mode.ctl" = enum16{"fs or Ts", "fs*M/N"}
  T55 = typedef "DSDLL Virtual Digitizer.lvlib/DSDLL Session.ctl" = cluster{"dsdll":T56, "channels":i32, "device id":i32, "channel idns":string[], "proc setup":T58, "samples count":i32, "fs [Hz]":dbl}
  T56 = typedef "dsdll.lvlib/dsdll_instance.ctl" = cluster{"dsdll path":path, "dsdll handle":u8[], "output devices":T57[], "capture devices":T57[]}
  T57 = typedef "dsdll.lvlib/dsdll_device_record.ctl" = cluster{"guid":u8[], "name":string}
  T58 = typedef "DSDLL Virtual Digitizer.lvlib/DSDLL Process Config.ctl" = cluster{"packet size [smpl]":i32, "current timeout [s]":dbl, "blk2blk timeout [s]":dbl, "event time":timestamp, "data queue":refnum<queue>, "stop notifier":refnum<notifier>, "proc ref":refnum<vi>}
  T59 = typedef "ADC Type.ctl" = enum16{"niScope", "3458A", "DirectSound DLL", "Keysight DSO", "cDAQ ADC", "CMI ADS127L21", "dummy"}
  T60 = typedef "SimAdc Config.ctl" = cluster{"channels":T61[], "range [V]":dbl, "Ts step [s]":dbl, "time [s]":dbl, "fs [Hz]":dbl, "count":i64, "smpl offset":i64, "set count":i64, "bit res":i32}
  T61 = typedef "SimAdc Channel Cfg.ctl" = cluster{"harmonics":dbl[][], "btn clear":bool, "noise":dbl, "fundamental [Hz]":dbl}
  T62 = typedef "ADC On Close Action.ctl" = enum16{"Immediate reset", "Delayed reset"}
  T63 = typedef "MPX Session.ctl" = cluster{"Type":T64, "gen com ssn":T65, "delay before [s]":dbl, "delay post [s]":dbl, "sequence":string[], "enabled":bool, "ref timestamp [s]":dbl, "idn string":string, "dev niScope":refnum<k15>, "niScope idx":i32, "QPMX ssn":T69, "VISA mux ssn":T72}
  T64 = typedef "MPX Type.ctl" = enum16{"Dummy", "Generic - COM port", "Generic - niScope PFI", "Generic - VISA commands", "QPMX"}
  T65 = typedef "GCOMM Session.ctl" = cluster{"visa":refnum<visa-resource-name>, "primary":T66, "secondary":T66, "channels":T67[]}
  T66 = typedef "GCOMM Signal.ctl" = enum16{"None", "DTR", "RTS"}
  T67 = typedef "GCOMM Virtual Channel.ctl" = cluster{"Primary:":T68, "Secondary:":T68, "btn clr":bool, "btn up":bool, "btn down":bool, "Tag:":string}
  T68 = typedef "GCOMM Logic State.ctl" = enum16{"OFF", "ON"}
  T69 = typedef "QPMX Session.ctl" = cluster{"visa":refnum<visa-resource-name>, "switch mode":T70, "sequence":bool[][], "timing delays":u32[], "polarity":T71, "ss delay (s)":dbl, "internal timer (s)":dbl, "Last loaded sequence file":path, "startup delay (s)":dbl}
  T70 = typedef "QPMX switch mode.ctl" = enum16{"Switched by TWM", "Switched by external clock", "Switched by internal clock"}
  T71 = typedef "QPMX polarity.ctl" = enum16{"Positive", "Negative"}
  T72 = typedef "GVISA Mux Session.ctl" = cluster{"VISA":refnum<visa-resource-name>, "paths":T73[], "idn command":string, "serial cfg":T74}
  T73 = typedef "GVISA Mux Path Entry.ctl" = cluster{"Tag:":string, "Command:":string, "btn clr":bool, "btn up":bool, "btn down":bool}
  T74 = typedef "met_serial_setup.ctl" = cluster{"Baud rate":i32, "Data bits":i32, "Parity":i32, "Stop bits":i32, "Flow control":i32, "End Mode Read":enum16{"None", "Last Bit", "TermChar"}, "End Mode Write":enum16{"None", "Last Bit", "TermChar"}, "Term character":u8, "Term enable":bool}
  T75 = typedef "KeDSO session.ctl" = cluster{"VISA":refnum<visa-resource-name>, "channels":T76[], "bw limit [Hz]":dbl, "resolution":T77, "trig noise reject":enum16{"Normal", "High Sensitivity"}, "N":i64, "trigger config":T78, "fs [Hz]":dbl, "timeout stop":timestamp, "waiting for opc":bool, "fetch offset [smpl]":i64, "abs timestamp":timestamp, "ranges [V]":dbl[], "decimation":dbl, "ext ref":bool, "emulate aperture":bool, "model":T80}
  T76 = typedef "KeDSO Virtual Channel.ctl" = cluster{"Channel":i32, "Range [Vpk]":dbl, "btn clr":bool, "btn up":bool, "btn down":bool, "Offset [V]":dbl, "Coupling":enum16{"DC", "DC50", "AC", "LFR1"}, "bw limit enab":bool}
  T77 = typedef "KeDSO High Resolution Mode.ctl" = enum16{"Basic", "High-res AUTO", "Min. 9-bits", "Min. 10-bits", "Min. 11-bits", "Min. 12-bits", "Fixed 11-bits", "Fixed 12-bits", "Fixed 13-bits", "Fixed 14-bits", "Fixed 15-bits", "Fixed 16-bits"}
  T78 = typedef "KeDSO Trigger Setup.ctl" = cluster{"trigger source":T79, "trigger slope":enum16{"Negative", "Positive", "Either"}, "level [V]":dbl, "hysteresis [V]":dbl, "pre-trig [%]":i32}
  T79 = typedef "KeDSO Trigger Source.ctl" = enum16{"Immediate", "Level", "AUX"}
  T80 = typedef "Agilent 90000 Series.lvlib/DSO type.ctl" = enum16{"DSO91304", "DSO91204", "DSO90804", "DSO90604", "DSO90404", "DSO90254", "DSA91304", "DSA91204", "DSA90804", "DSA90604", "DSA90404", "DSA90254", "DSO9104", "DSO9254", "DSO9404", "MSO9104", "MSO9254", "MSO9404", "MSO9064", "DSO9064", "DSOX91604", "DSOX92004", "DSOX92504", "DSOX92804", "DSOX93204", "DSO93004", "DSO9024H", "DSO9054H", "DSO9104H", "DSO9204H", "DSOS054A", "DSOS104A", "DSOS204A", "DSOS254A", "DSOS404A", "DSOS604A", "DSOS804A", "MSOS054A", "MSOS104A", "MSOS204A", "MSOS254A", "MSOS404A", "MSOS604A", "MSOS804A", "DSAX96204Q", "DSOX96204Q", "DSAX95004Q", "DSOX95004Q", "DSAX93304Q", "DSOX93304Q", "DSAX92504Q", "DSOX92504Q", "DSAX92004Q", "DSOX92004Q"}
  T81 = typedef "cDAQ Session.ctl" = cluster{"mclk [Hz]":dbl, "ADC task":refnum<k21>, "mclk reference":string, "fs [Hz]":dbl, "queue adc cmd":refnum<queue>, "queue adc data":refnum<queue>, "adc proc ref":refnum<vi>, "channels":T82[], "last channels":T82[], "timeout":timestamp, "N":i32, "mclk mode":T83, "ext mclk source":tag}
  T82 = typedef "cDAQ Virtual Channel.ctl" = cluster{"Device":tag, "Channel id":i32, "btn clr":bool, "btn up":bool, "btn down":bool}
  T83 = typedef "cDAQ Master Clock Mode.ctl" = enum16{"Free running", "Export master clock", "Import master clock"}
  T84 = typedef "CMI ADS127L21 - Session.ctl" = cluster{"VISA":refnum<visa-resource-name>, "chn list":i32[], "record size":i32, "phys. channels":i32, "adc fifo size":i32, "channels":T85[], "ext refclk?":bool, "fs [Hz]":dbl, "ext refclk [Hz]":dbl, "meas refclk [Hz]":dbl, "EXTOUT mode":T89, "EXTOUT polarity":T90, "EXTOUT divisor":i32}
  T85 = typedef "CMI ADS127L21 - Record Channel.ctl" = cluster{"Range [Vpk]":T86, "Channel":i32, "Mode":T87, "Impedance":T88, "btn clr":bool, "btn up":bool, "btn down":bool}
  T86 = typedef "CMI ADS127L21 - Input Range.ctl" = dbl
  T87 = typedef "CMI ADS127L21 - Input Mode.ctl" = enum16{"Normal", "Inverted", "GND"}
  T88 = typedef "CMI ADS127L21 - Input Impedance.ctl" = enum16{"1M", "1k5"}
  T89 = typedef "CMI ADS127L21 - EXTOUT Mode.ctl" = enum16{"ADCCLK", "REFCLK", "SMPLCLK", "FIRST"}
  T90 = typedef "CMI ADS127L21 - EXTOUT Polarity.ctl" = enum16{"NORM", "INV"}
  T91 = typedef "Meas Session.ctl" = cluster{"adc":T7, "sequence":T92[], "sequence setup":T95, "golpi":T96, "processing setup":T97, "corrections":T107, "assist cfg":T110}
  T92 = typedef "Meas Sequence Item.ctl" = cluster{"config":T93, "data file path":path, "header file path":path, "group id":i32, "rec id":i32, "group done?":bool, "adc modified?":bool, "source modified?":bool, "progress [%]":dbl, "groups cnt":i32, "rec cnt":i32, "data file relative path":string, "meas root path":path, "calculate?":bool, "comment":string, "avg cnt":i32}
  T93 = typedef "Meas Sampling Configuration.ctl" = cluster{"count [smpl]":i64, "aperture [s]":dbl, "trigger":T37, "ranges [Vpk]":dbl[], "QWTB parameters":T94[], "sampling rate":T52}
  T94 = typedef "Meas Proc QWTB Algorithm Parameter Data.ctl" = cluster{"name":string, "numerics":dbl[], "strings":string[]}
  T95 = typedef "Meas Sequence Configuration.ctl" = cluster{"group setups":T93[], "rec count":i32, "range mode":T3, "fs mode":T2, "rng even":dbl, "rng odd":dbl, "folder":path, "name base":string, "meas id":i32, "settle [s]":dbl, "comment":string, "avg count":i32, "fs-abs-fr fr":dbl, "fs-abs-fr fs":dbl, "fs-div fr":dbl, "fs-div div":dbl, "fs-mn fr":dbl, "fs-mn mul":dbl, "fs-mn div":dbl, "fs-rat fr":dbl, "fs-rat rat":dbl}
  T96 = typedef "GOLPI Multi Process.lvlib/golpi_session_ref.ctl" = refnum<vi>
  T97 = typedef "Meas Process Config.ctl" = cluster{"mode":T98, "call after avgs?":bool, "calculate?":bool, "raw mode":T99, "QWTB":T101}
  T98 = typedef "Meas Process Mode.ctl" = enum16{"Raw", "QWTB"}
  T99 = typedef "Meas Process Raw Config.ctl" = cluster{"command":string, "result mode":T100, "res variable":string}
  T100 = typedef "Meas Process Raw Result Mode.ctl" = enum16{"Display console output (only Octave)", "Display string variable", "Display result file %respath%"}
  T101 = typedef "Meas Proc QWTB Setup.ctl" = cluster{"QWTB path":path, "alg filter path":string, "alg ids":string[], "alg parameters":string[], "parsed parameters":T94[], "selected alg id":string, "selected unc mode":T102, "qwtb mcc":i32, "qwtb timeout":i32, "qwtb covg":dbl, "qwtb ofs":i64, "qwtb lim data":i64, "multicore":T103, "unc once?":bool, "qwtb tstemp":T105, "octave reset":bool, "exec mode":T106}
  T102 = typedef "Meas Proc QWTB Uncertainty Mode.ctl" = enum16{"None", "GUF", "Monte Carlo"}
  T103 = typedef "Meas Proc QWTB Multicore Setup.ctl" = cluster{"jobs folder":path, "cores":i32, "max jobs":i32, "mode":T104}
  T104 = typedef "Meas Proc QWTB Multicore Type.ctl" = enum16{"Singlecore", "Multicore", "Multistation"}
  T105 = typedef "Meas Process Time Stamp Mode.ctl" = enum16{"Enabled (default)", "Disabled", "Relative to 1. record"}
  T106 = typedef "Meas Proc QWTB Exec Mode.ctl" = enum16{"Single-core", "Parallel Record Processing"}
  T107 = typedef "Corr Setup.ctl" = cluster{"transducers":cluster{"channels":T108[], "last path":path, "root path":path}, "digitizer":T109}
  T108 = typedef "Corr Tranducer Item.ctl" = cluster{"Path":path, "Ratio:":string, "Name:":string, "btn rem":bool, "btn up":bool, "btn down":bool, "s.n.:":string, "btn open":bool, "ratio o/i":dbl, "chn hi":u16, "chn lo":u16, "Phase index":i32, "btn edit":bool, "mpx chn":u16, "btn vdx1":bool, "btn csx1":bool, "invert":bool}
  T109 = typedef "Corr Digitizers.ctl" = cluster{"last path":path, "channel paths":path[], "channel idns":string[], "correction name":string, "channel names":string[], "folders to copy":path[], "channel valid":bool[], "correction path":path, "correction rel path":string, "rel folders to copy":string[], "root path":path}
  T110 = typedef "Assist Panel Setup.ctl" = cluster{"P":i32, "Q":i32, "rel shift":dbl, "ref freq":dbl, "min fs":dbl, "max fs tol":dbl, "min int":dbl, "max int":dbl, "max err":dbl, "max timeout":dbl}
  T111 = typedef "GUI Panel Control Action.ctl" = enum16{"Open panel", "Close panel", "Bring To Front"}
  T112 = typedef "varilib.lvlib/SGUI Assign References Mode.ctl" = enum16{"Add to stack", "Overwrite", "Release last", "Release ID"}
  T113 = typedef "ADC Capabilities Parameters.ctl" = cluster{"fs [Hz]":dbl, "aperture [s]":dbl}
  T114 = enum32{"abs", "abs fr", "fr/N", "fr*M/N", "fr*R", "fix"}[]
  T115 = typedef "ADC Capabilities.ctl" = cluster{"max samples count":i64, "max fs [Hz]":ext, "min fs [Hz]":ext, "Ts step [s]":ext, "max Ts [s]":ext, "min Ts [s]":ext, "allows streaming?":bool, "streaming on?":bool, "has level trig?":bool, "has ext trig?":bool, "has aperture?":bool, "aper min [s]":dbl, "aper max [s]":dbl, "channels count":i32, "has ranges?":bool, "has temperature?":bool, "has temperature log?":bool, "has selfcal?":bool, "fs step [Hz]":ext, "smpl rate step mode":T116, "no aper info":string, "no fs info":string, "has fs?":bool, "srate mode":T53, "auto aperture?":bool, "auto aperture [s]":ext, "user fs mode option?":bool, "has pre-trigger?":bool, "has trigger hyst?":bool}
  T116 = typedef "ADC Sampling Rate Step Mode.ctl" = enum16{"const period", "const frequency"}
  T117 = typedef "Assist Sampling Setup.ctl" = cluster{"fs [Hz]":ext, "N":i64, "error":dbl}
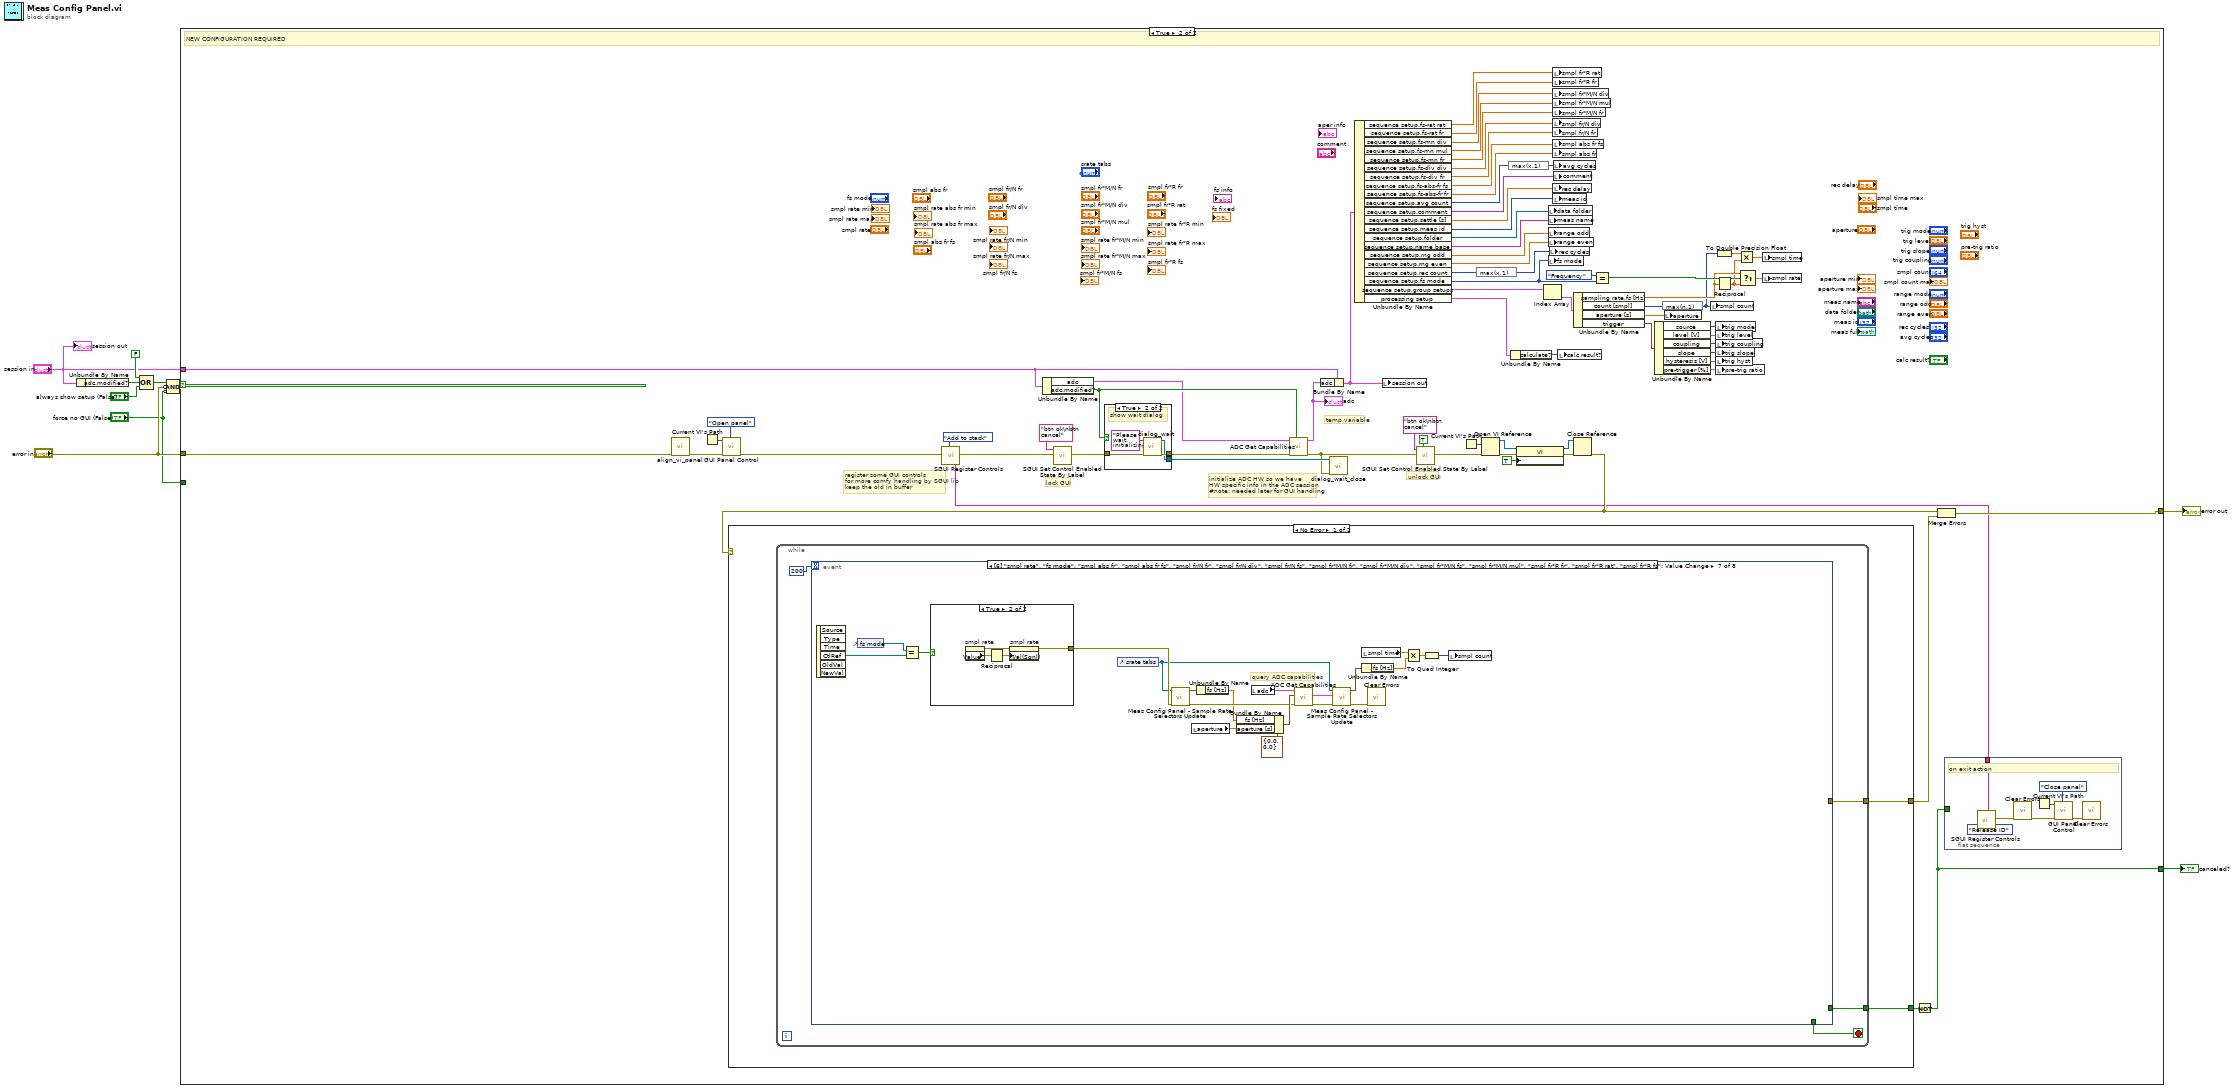
[diagram p0: block diagram]
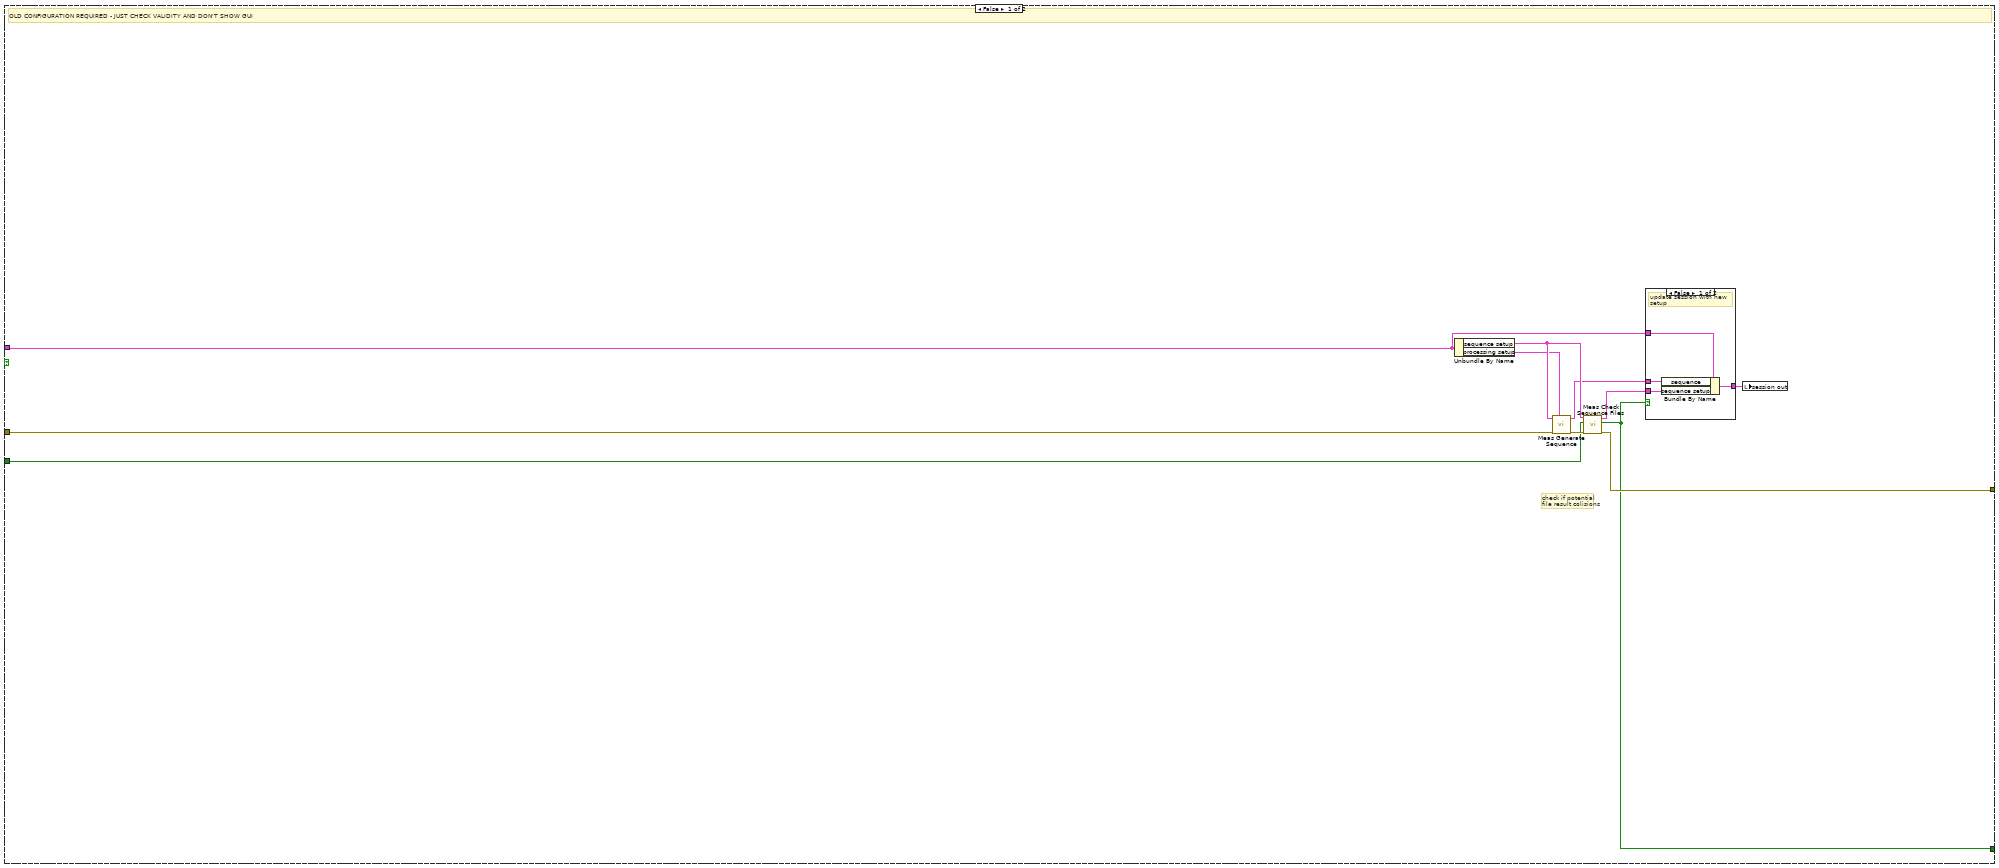
[diagram p2: hidden frame]
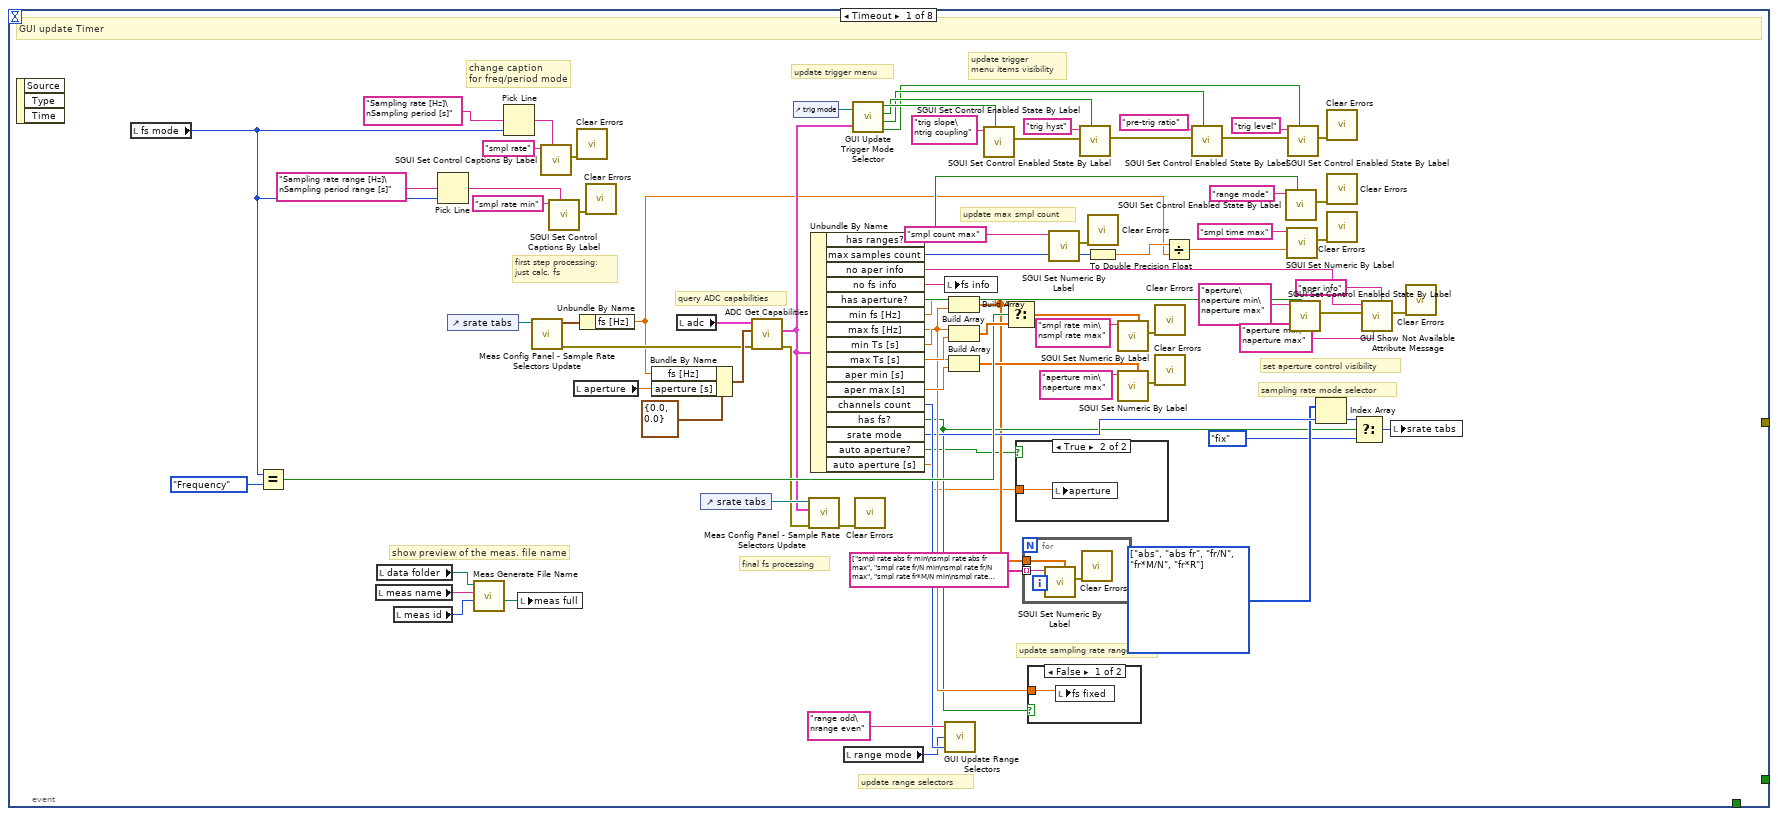
[diagram p5: hidden frame]
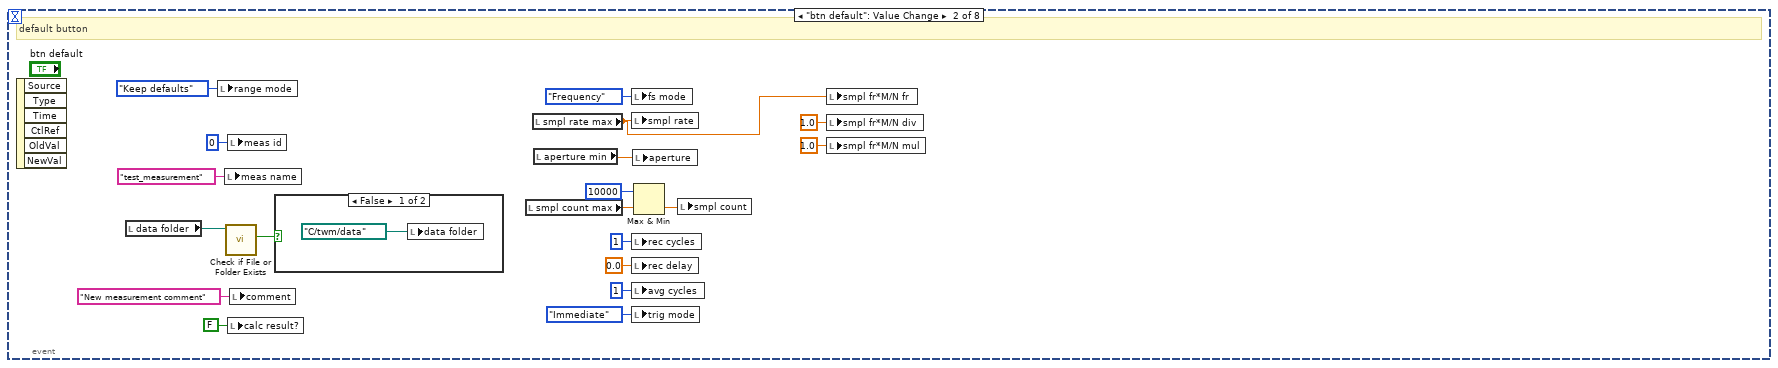
[diagram p8: hidden frame]
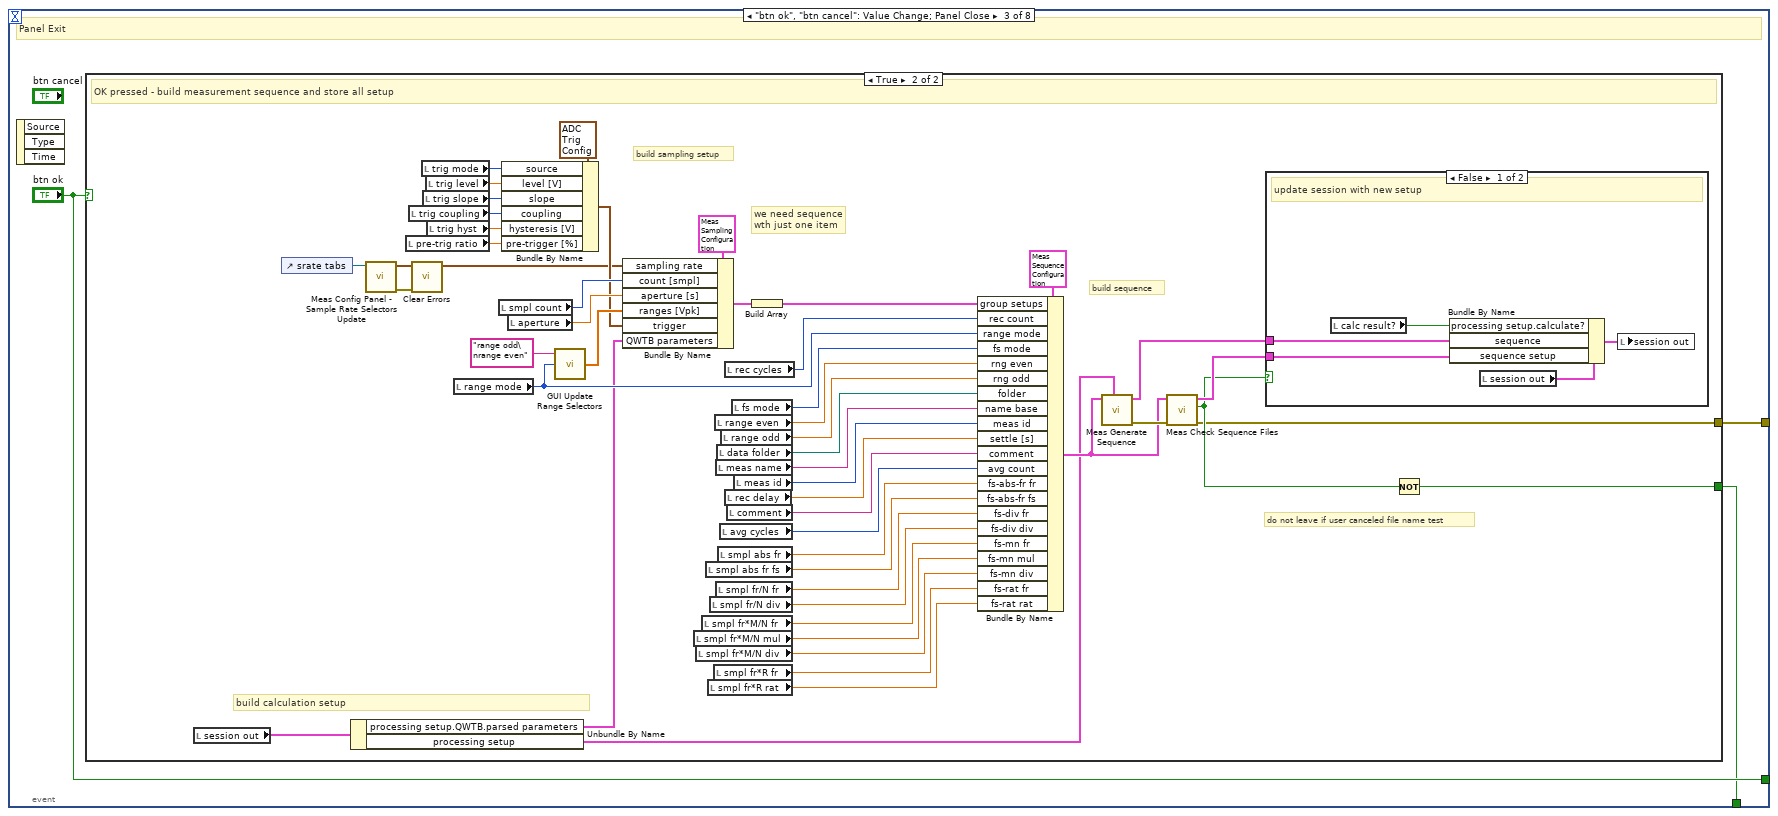
[diagram p10: hidden frame]
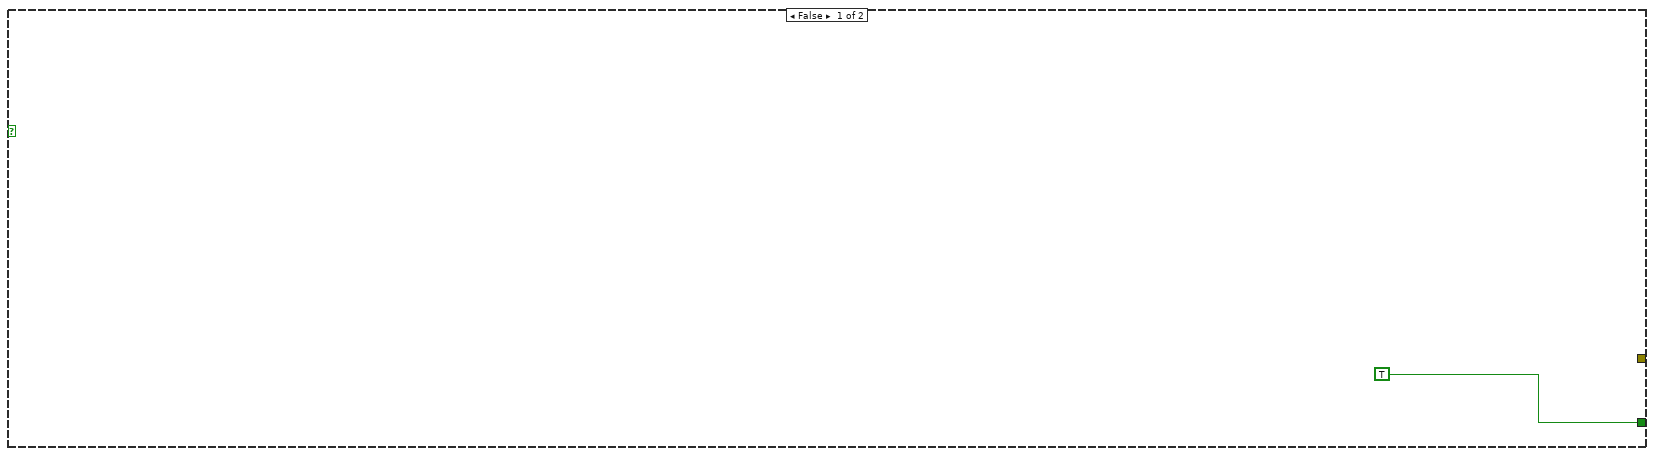
[diagram p11: hidden frame]
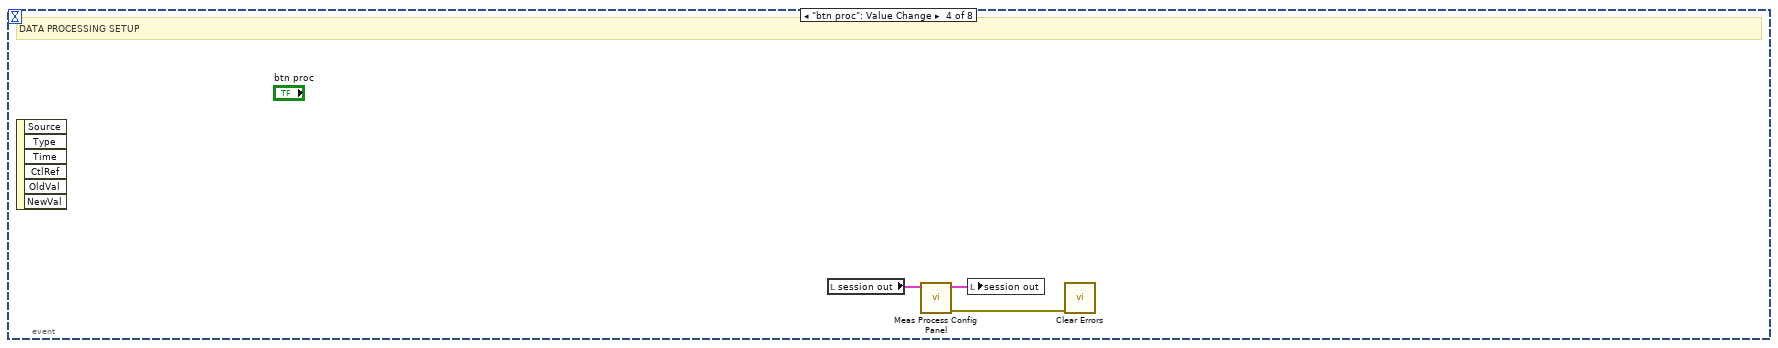
[diagram p13: hidden frame]
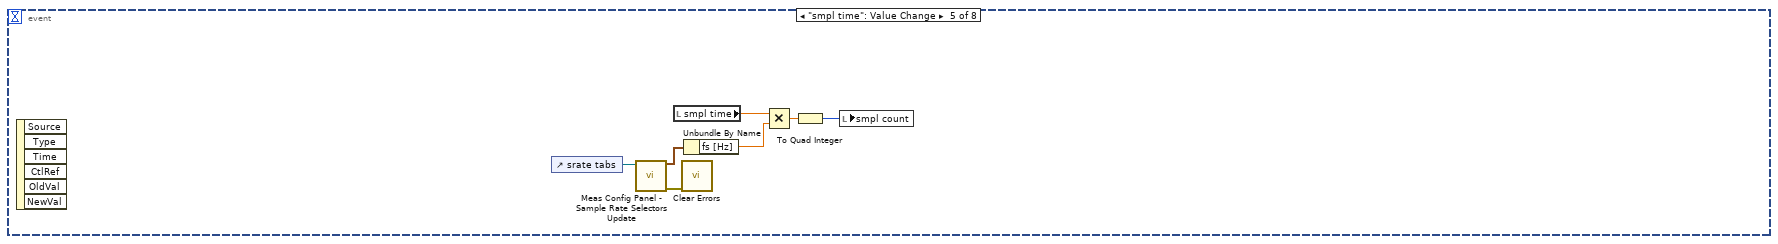
[diagram p14: hidden frame]
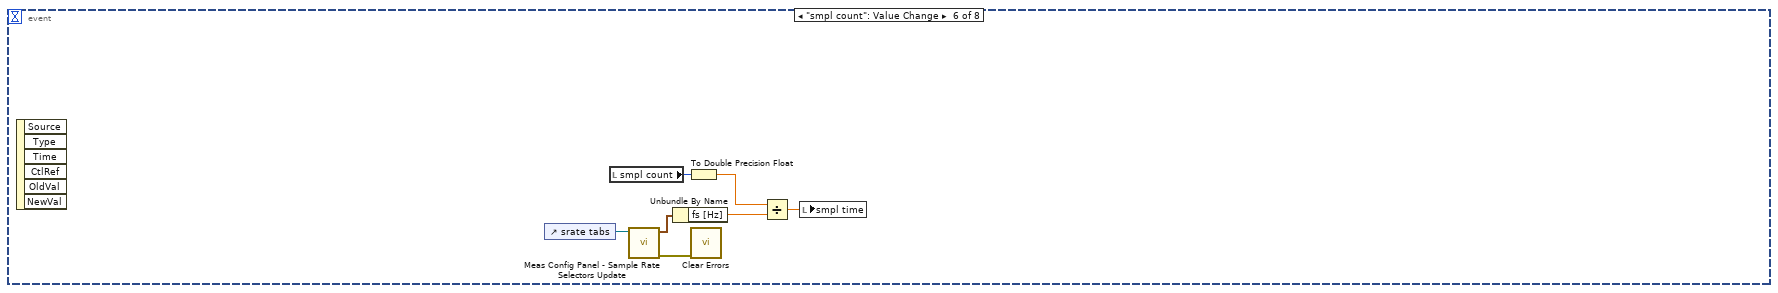
[diagram p15: hidden frame]
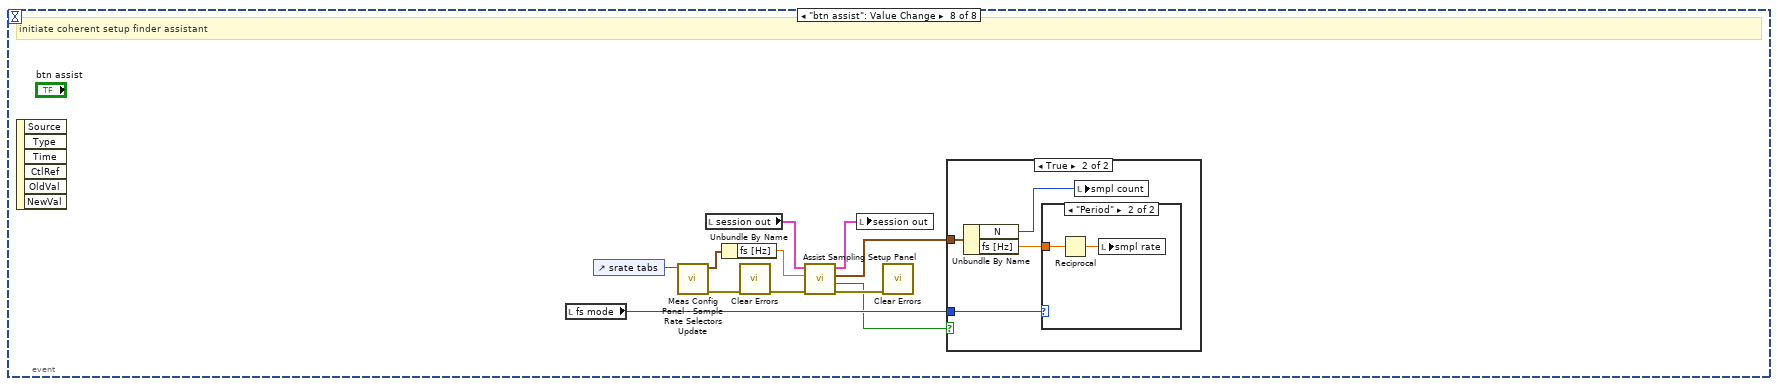
[diagram p17: hidden frame]
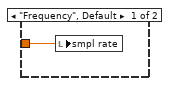
[diagram p19: hidden frame]
diagram:
  n1 = Unbundle By Name("session in") -> ("adc.modified?"=w9:bool)
  n2 = Compound Arithmetic op=OR(FALSE ("value"), w9, "always show setup (False)") -> (w7:bool)
  n3 = Compound Arithmetic op=AND(w7, invert "error in", invert "force no GUI (False)") -> (w10:bool)
  n4 = case shown="True" w10 {
    tunnel: "error in" -> [w20 w71]
    tunnel: "session in" -> [w12 w63]
    tunnel: [w16 w55] -> w4
    tunnel: [w21 w47] -> w3
    tunnel: "force no GUI (False)" -> [w13 _]
    frame False {
      # "check if potential\nfile result colisions"
      # "OLD CONFIGURATION REQUIRED - JUST CHECK VALIDITY AND DON'T SHOW GUI"
      n5 = Unbundle By Name(w12) -> ("sequence setup"=w18:T95, "processing setup"=w17:T97)
      n6 = call "Meas Generate Sequence.vi"("processing setup"=w17, "error in"=w20, "sequence setup"=w18) -> ("error out"=w19:errorcluster, "sequence out"=w15:T92[])  [unwired: 6 in, 1 out]
      n7 = call "Meas Check Sequence Files.vi"("error in"=w19, "don't ask (False)"=w13, "sequence setup"=w18) -> ("error out"=w21:errorcluster, "cancel?"=w16:bool, "sequence setup out (copy)"=w14:T95)  [unwired: 6 in]
      n8 = case shown="False" w16 {
        tunnel: w15 -> [w25 _]
        tunnel: w14 -> [w24 _]
        tunnel: w12 -> [w23 w26]
        tunnel: [w22 w26] -> w11
        frame False {
          # "update session with new setup"
          n9 = Bundle By Name(cluster=w23, "sequence"=w25, "sequence setup"=w24) -> (w22:T91)
        }
        frame True {
        }
      }
      n10 = local write "session out"(w11) -> ()
    }
    frame True {
      # "unlock GUI"
      # "lock GUI"
      # "temp variable"
      # "register some GUI controls\nfor more comfy handling by SGUI lib\nkeep the old in buffer"
      # "initialize ADC HW so we have\nHW specific info in the ADC session\n#note: needed later for GUI handling"
      # "NEW CONFIGURATION REQUIRED"
      n11 = call "align_vi_panel.vi"("error in"=w71) -> ("error out"=w60:errorcluster)  [unwired: 10 in]
      n12 = Current VI's Path() -> (path=w58:path)
      n13 = call "GUI Panel Control.vi"("action (open panel)"=GUI_Panel_Control_Action."Open panel", "error in (no error)"=w60, "vi path"=w58) -> ("error out"=w59:errorcluster)  [unwired: 8 in]
      n14 = call "SGUI Register Controls.vi"("error in"=w59, "register mode (overwrite)"=SGUI_Assign_References_Mode."Add to stack") -> ("assigned ID"=w46:string, "error out"=w79:errorcluster)  [unwired: 15 in, 1 out]
      n15 = Unbundle By Name(w63) -> ("adc"=w44:T7, "adc.modified?"=w76:bool)
      n16 = call "SGUI Set Control Enabled State By Label.vi"("error in"=w79, "labels (empty)"="btn ok\nbtn cancel") -> ("error out"=w77:errorcluster)  [unwired: 8 in, 1 out]
      n17 = case shown="True" w76 {
        tunnel: w77 -> [w101 w105]
        tunnel: [w101 w104] -> w45
        tunnel: [_ w102] -> w75
        frame False {
        }
        frame True {
          # "show wait dialog"
          n18 = call "dialog_wait.vi"("error in"=w105, "message string"="Please wait, initializing HW ...") -> ("error out"=w104:errorcluster, "reference out"=w102:refnum<vi>)  [unwired: 8 in]
        }
      }
      n19 = call "ADC Get Capabilities.vi"("Initialize HW? (False)"=w76, "error in"=w45, "adc session in"=w44) -> ("error out"=w74:errorcluster, "adc session out"=w100:T7)  [unwired: 6 in, 1 out]
      "adc" <- w100
      n20 = Bundle By Name(cluster=w63, "adc"=w100) -> (w54:T91)
      n21 = call "dialog_wait_close.vi"("error in"=w74, "async vi ref"=w75) -> ()  [unwired: 2 in]
      n22 = Unbundle By Name(w54) -> ("sequence setup.fs-rat rat"=w32:dbl, "sequence setup.fs-rat fr"=w33:dbl, "sequence setup.fs-mn div"=w34:dbl, "sequence setup.fs-mn mul"=w35:dbl, "sequence setup.fs-mn fr"=w36:dbl, "sequence setup.fs-div div"=w37:dbl, "sequence setup.fs-div fr"=w38:dbl, "sequence setup.fs-abs-fr fs"=w39:dbl, "sequence setup.fs-abs-fr fr"=w40:dbl, "sequence setup.avg count"=w41:i32, "sequence setup.comment"=w42:string, "sequence setup.settle [s]"=w43:dbl, "sequence setup.meas id"=w56:i32, "sequence setup.folder"=w81:path, "sequence setup.name base"=w82:string, "sequence setup.rng odd"=w83:dbl, "sequence setup.rng even"=w84:dbl, "sequence setup.rec count"=w94:i32, "sequence setup.fs mode"=w92:T2, "sequence setup.group setups"=w98:T93[], "processing setup"=w65:T97)
      n23 = local write "session out"(w54) -> ()
      n24 = call "SGUI Set Control Enabled State By Label.vi"("error in"=w74, "labels (empty)"="btn ok\nbtn cancel", "Enabled? (False)"=TRUE) -> ("error out"=w67:errorcluster)  [unwired: 7 in, 1 out]
      n25 = Current VI's Path() -> (path=w70:path)
      n26 = expression code="max(x,1)"(w94) -> (w30:i32)
      n27 = Open VI Reference(vi path=w70, error in (no error)=w67) -> (vi reference=w69:refnum<vi>, error out=w68:errorcluster)  [unwired: 4 in]
      n28 = expression code="max(x,1)"(w41) -> (w31:i32)
      n29 = Unbundle By Name(w65) -> ("calculate?"=w64:bool)
      n30 = property class="VI"(reference=w69, error in=w68, "Front Panel.IsFrontmost"=TRUE ("Front Panel Window:Is Frontmost")) -> (reference out=w61:refnum<vi>, error out=w62:errorcluster)
      n31 = Index Array(array=w98) -> (element=w97:T93)  [unwired: 1 in]
      n32 = local write "data folder"(w81) -> ()
      n33 = local write "meas name"(w82) -> ()
      n34 = local write "range odd"(w83) -> ()
      n35 = local write "range even"(w84) -> ()
      n36 = local write "fs mode"(w92) -> ()
      n37 = local write "rec cycles"(w30) -> ()
      n38 = local write "smpl fr*R rat"(w32) -> ()
      n39 = local write "smpl fr*R fr"(w33) -> ()
      n40 = local write "smpl fr*M/N div"(w34) -> ()
      n41 = local write "smpl fr*M/N mul"(w35) -> ()
      n42 = local write "smpl fr*M/N fr"(w36) -> ()
      n43 = local write "smpl fr/N div"(w37) -> ()
      n44 = local write "smpl fr/N fr"(w38) -> ()
      n45 = local write "smpl abs fr fs"(w39) -> ()
      n46 = local write "smpl abs fr"(w40) -> ()
      n47 = local write "rec delay"(w43) -> ()
      n48 = local write "meas id"(w56) -> ()
      n49 = local write "avg cycles"(w31) -> ()
      n50 = local write "comment"(w42) -> ()
      n51 = local write "calc result?"(w64) -> ()
      n52 = Unbundle By Name(w97) -> ("sampling rate.fs [Hz]"=w95:dbl, "count [smpl]"=w50:i64, "aperture [s]"=w90:dbl, "trigger"=w89:T37)
      n53 = Close Reference(reference=w61, error in (no error)=w62) -> (error out=w49:errorcluster)
      n54 = case shown="No Error" w49 {
        tunnel: [w114 _] -> w99
        tunnel: [w113 _] -> w48
        frame No Error {
          n55 = while {
            tunnel: [w116] -> w114
            tunnel: [w115] -> w113
            stop <- w117 stop-if-true
            n56 = event shown="[6] \"smpl rate\", \"fs mode\", \"smpl abs fr\", \"smpl abs fr fs\", \"smpl fr/N fr\", \"smpl fr/N div\", \"smpl fr/N fs\", \"smpl fr*M/N fr\", \"smpl fr*M/N div\", \"smpl fr*M/N fs\", \"smpl fr*M/N mul\", \"smpl fr*R fr\", \"smpl fr*R rat\", \"smpl fr*R fs\": Value Change" {
              selector: _ -> [_ _ _ _ _ _ _ _]
              dyn-events: _ -> [_ _ _ _ _ _ _ _]
              timeout: 200 -> [_ _ _ _ _ _ _ _]
              tunnel: [_ _ w229 _ _ _ _ _] -> w117
              tunnel: [_ _ "btn ok" _ _ _ _ _] -> w116
              tunnel: [_ _ w228 _ _ _ _ _] -> w115
              event Timeout {
                w149 = T114 [enum."abs", enum."abs fr", enum."fr/N", enum."fr*M/N", enum."fr*R"] items=["abs", "abs fr", "fr/N", "fr*M/N", "fr*R", "fix"]
                # "final fs processing"
                # "first step processing:\njust calc. fs"
                # "sampling rate mode selector"
                # "show preview of the meas. file name"
                # "update range selectors"
                # "update sampling rate ranges"
                # "update max smpl count"
                # "update trigger\nmenu items visibility"
                # "update trigger menu"
                # "set aperture control visibility"
                # "query ADC capabilities"
                # "change caption\nfor freq/period mode"
                # "GUI update Timer"
                n57 = event-data() -> ()  [unwired: 1 in, 3 out]
                n58 = local read "fs mode"() -> (w129:T2)
                n59 = Equal?(x=w129, y=Meas_Sampling_Rate_Mode."Frequency") -> (x = y?=w185:bool)
                n60 = local read "meas name"() -> (w165:string)
                n61 = local read "data folder"() -> (w163:path)
                n62 = local read "meas id"() -> (w164:i32)
                n63 = Pick Line(multi-line string="Sampling rate range [Hz]\nSampling period range [s]", line index=w129) -> (output string=w135:string)  [unwired: 1 in]
                n64 = control-ref of="srate tabs"() -> (w134:refnum<vi>)
                n65 = call "Meas Generate File Name.vi"("meas id"=w164, "name base"=w165, "folder"=w163) -> ("header file full path"=w162:path)  [unwired: 4 in, 4 out]
                n66 = Pick Line(multi-line string="Sampling rate [Hz]\nSampling period [s]", line index=w129) -> (output string=w200:string)  [unwired: 1 in]
                n67 = local write "meas full"(w162) -> ()
                n68 = call "Meas Config Panel - Sample Rate Selectors Update.vi"("tab control ref"=w134) -> ("error out"=w133:errorcluster, "sampling rate"=w132:T52)  [unwired: 9 in]
                n69 = call "SGUI Set Control Captions By Label.vi"("labels (empty)"="smpl rate", "captions (empty)"=w200) -> ("error out"=w173:errorcluster)  [unwired: 8 in, 1 out]
                n70 = call "SGUI Set Control Captions By Label.vi"("labels (empty)"="smpl rate min", "captions (empty)"=w135) -> ("error out"=w172:errorcluster)  [unwired: 8 in, 1 out]
                n71 = local read "aperture"() -> (w193:dbl)
                n72 = call <vilib>:"Clear Errors.vi"("error in (no error)"=w173) -> ()  [unwired: 5 in, 2 out]
                n73 = Unbundle By Name(w132) -> ("fs [Hz]"=w131:dbl)
                n74 = call <vilib>:"Clear Errors.vi"("error in (no error)"=w172) -> ()  [unwired: 5 in, 2 out]
                n75 = Bundle By Name(cluster=T113 {"fs [Hz]"=0.0, "aperture [s]"=0.0} ("parameters"), "fs [Hz]"=w131, "aperture [s]"=w193) -> (w197:T113)
                n76 = local read "adc"() -> (w199:T7)
                n77 = control-ref of="srate tabs"() -> (w140:refnum<vi>)
                n78 = call "ADC Get Capabilities.vi"("error in"=w133, "parameters"=w197, "adc session in"=w199) -> ("error out"=w130:errorcluster, "capabilities"=w136:T115)  [unwired: 6 in, 1 out]
                n79 = control-ref of="trig mode"() -> (w192:refnum<vi>)
                n80 = call "Meas Config Panel - Sample Rate Selectors Update.vi"("error in (no error)"=w130, "adc capabilities"=w136, "tab control ref"=w140) -> ("error out"=w139:errorcluster)  [unwired: 7 in, 1 out]
                n81 = Unbundle By Name(w136) -> ("has ranges?"=w166:bool, "max samples count"=w161:i64, "no aper info"=w152:string, "no fs info"=w141:string, "has aperture?"=w194:bool, "min fs [Hz]"=w189:ext, "max fs [Hz]"=w151:ext, "min Ts [s]"=w188:ext, "max Ts [s]"=w187:ext, "aper min [s]"=w181:dbl, "aper max [s]"=w180:dbl, "channels count"=w170:i32, "has fs?"=w148:bool, "srate mode"=w150:T53, "auto aperture?"=w138:bool, "auto aperture [s]"=w137:ext)
                n82 = local read "range mode"() -> (w169:T3)
                n83 = call "GUI Update Trigger Mode Selector.vi"("trig mode ref"=w192, "capabilities"=w136) -> ("has parameters?"=w190:bool, "has hysteresis?"=w125:bool, "has pre-trigger?"=w121:bool, "has level?"=w119:bool)
                n84 = call <vilib>:"Clear Errors.vi"("error in (no error)"=w139) -> ()  [unwired: 5 in, 2 out]
                n85 = local write "fs info"(w141) -> ()
                n86 = call "GUI Update Range Selectors.vi"("total channels"=w170, "range mode"=w169, "odd and even item names"="range odd\nrange even") -> ()  [unwired: 1 out]
                n87 = Build Array(w189, w151) -> (w142:ext[])
                n88 = Build Array(w188, w187) -> (w186:ext[])
                n89 = Build Array(w181, w180) -> (w178:dbl[])
                n90 = call "SGUI Set Control Enabled State By Label.vi"("labels (empty)"="trig slope\ntrig coupling", "Enabled? (False)"=w190) -> ("error out"=w124:errorcluster)  [unwired: 8 in, 1 out]
                n91 = Select(t=w142, s=w185, f=w186) -> (s? t:f=w183:ext[])
                n92 = case shown="True" w138 {
                  tunnel: w137 -> [_ w203]
                  frame False {
                  }
                  frame True {
                    n93 = local write "aperture"(w203) -> ()
                  }
                }
                n94 = for {
                  tunnel: string[] ["smpl rate abs fr min\nsmpl rate abs fr max", "smpl rate fr/N min\nsmpl rate fr/N max", "smpl rate fr*M/N min\nsmpl rate fr*M/N max", "smpl rate fr*R min\nsmpl rate fr*R max"] -> [w205] mode=indexing
                  tunnel: w142 -> [w204]
                  n95 = call-poly "SGUI Set Numeric By Label.vi"("labels (empty)"=w205, "numbers (empty)"=w204) -> ("error out"=w206:errorcluster)  [unwired: 8 in, 1 out]
                  n96 = call <vilib>:"Clear Errors.vi"("error in (no error)"=w206) -> ()  [unwired: 5 in, 2 out]
                }
                n97 = case shown="False" w148 {
                  tunnel: w151 -> [w207 _]
                  frame False {
                    n98 = local write "fs fixed"(w207) -> ()
                  }
                  frame True {
                  }
                }
                n99 = call-poly "SGUI Set Numeric By Label.vi"("label (empty)"="smpl count max" ("labels (empty)"), "value (none)"=w161) -> ("error out"=w176:errorcluster)  [unwired: 8 in, 1 out]
                n100 = call "SGUI Set Control Enabled State By Label.vi"("error in"=w124, "labels (empty)"="trig hyst", "Enabled? (False)"=w125) -> ("error out"=w122:errorcluster)  [unwired: 7 in, 1 out]
                n101 = call <vilib>:"Clear Errors.vi"("error in (no error)"=w176) -> ()  [unwired: 5 in, 2 out]
                n102 = To Double Precision Float(number=w161) -> (double precision float=w157:dbl)
                n103 = call-poly "SGUI Set Numeric By Label.vi"("labels (empty)"="smpl rate min\nsmpl rate max", "numbers (empty)"=w183) -> ("error out"=w175:errorcluster)  [unwired: 8 in, 1 out]
                n104 = call-poly "SGUI Set Numeric By Label.vi"("labels (empty)"="aperture min\naperture max", "numbers (empty)"=w178) -> ("error out"=w174:errorcluster)  [unwired: 8 in, 1 out]
                n105 = call <vilib>:"Clear Errors.vi"("error in (no error)"=w175) -> ()  [unwired: 5 in, 2 out]
                n106 = call <vilib>:"Clear Errors.vi"("error in (no error)"=w174) -> ()  [unwired: 5 in, 2 out]
                n107 = Divide(x=w157, y=w131) -> (x/y=w160:dbl)
                n108 = call "SGUI Set Control Enabled State By Label.vi"("error in"=w122, "labels (empty)"="pre-trig ratio", "Enabled? (False)"=w121) -> ("error out"=w120:errorcluster)  [unwired: 7 in, 1 out]
                n109 = call "SGUI Set Control Enabled State By Label.vi"("labels (empty)"="range mode", "Enabled? (False)"=w166) -> ("error out"=w168:errorcluster)  [unwired: 8 in, 1 out]
                n110 = call-poly "SGUI Set Numeric By Label.vi"("label (empty)"="smpl time max", "value (none)"=w160) -> ("error out"=w158:errorcluster)  [unwired: 8 in, 1 out]
                n111 = call "SGUI Set Control Enabled State By Label.vi"("error in"=w120, "labels (empty)"="trig level", "Enabled? (False)"=w119) -> ("error out"=w126:errorcluster)  [unwired: 7 in, 1 out]
                n112 = call "SGUI Set Control Enabled State By Label.vi"("labels (empty)"="aperture\naperture min\naperture max", "Enabled? (False)"=w194) -> ("error out"=w156:errorcluster)  [unwired: 8 in, 1 out]
                n113 = Index Array(array=w149, index=w150) -> (element=w147:T1)
                n114 = call <vilib>:"Clear Errors.vi"("error in (no error)"=w126) -> ()  [unwired: 5 in, 2 out]
                n115 = call <vilib>:"Clear Errors.vi"("error in (no error)"=w168) -> ()  [unwired: 5 in, 2 out]
                n116 = call <vilib>:"Clear Errors.vi"("error in (no error)"=w158) -> ()  [unwired: 5 in, 2 out]
                n117 = Select(t=w147, s=w148, f=T1."fix") -> (s? t:f=w144:T1)
                n118 = call "GUI Show Not Available Attribute Message.vi"("SGUI info control label (none)"="aper info", "SGUI control lablels to disable (empty)"="aperture min\naperture max" ("labels (empty)"), "error in"=w156, "disabled message (empty)"=w152) -> ("error out"=w153:errorcluster)  [unwired: 7 in]
                n119 = local write "srate tabs"(w144) -> ()
                n120 = call <vilib>:"Clear Errors.vi"("error in (no error)"=w153) -> ()  [unwired: 5 in, 2 out]
              }
              event "btn default": Value Change {
                # "default button"
                n121 = event-data() -> ()  [unwired: 1 in, 6 out]
                n122 = local read "data folder"() -> (w223:path)
                n123 = local write "range mode"(Meas_Range_Mode."Keep defaults" ("range mode")) -> ()
                n124 = local write "meas name"("test_measurement" ("meas name")) -> ()
                n125 = call <vilib>:"Check if File or Folder Exists.vi"("path"=w223) -> ("file or folder exists?"=w222:bool)  [unwired: 8 in, 2 out]
                n126 = local write "meas id"(0 ("meas id")) -> ()
                n127 = local write "calc result?"(FALSE ("calc result?")) -> ()
                n128 = local write "comment"("New measurement comment" ("comment")) -> ()
                n129 = case shown="False" w222 {
                  frame False {
                    n130 = local write "data folder"(path "C:/twm/data" ("data folder")) -> ()
                  }
                  frame True {
                  }
                }
                n131 = local read "smpl count max"() -> (w216:dbl)
                n132 = local read "smpl rate max"() -> (w208:dbl)
                n133 = local read "aperture min"() -> (w218:dbl)
                n134 = local write "fs mode"(Meas_Sampling_Rate_Mode."Frequency" ("fs mode")) -> ()
                n135 = local write "smpl rate"(w208) -> ()
                n136 = local write "rec cycles"(1 ("rec cycles")) -> ()
                n137 = local write "rec delay"(0.0 ("rec delay")) -> ()
                n138 = local write "avg cycles"(1 ("avg cycles")) -> ()
                n139 = local write "trig mode"(ADC_Trig_Mode_Source."Immediate" ("trig mode")) -> ()
                n140 = local write "aperture"(w218) -> ()
                n141 = Max & Min(x=i64 10000 ("smpl count"), y=w216) -> (min(x,y)=w215:dbl)  [unwired: 1 out]
                n142 = local write "smpl count"(w215) -> ()
                n143 = local write "smpl fr*M/N fr"(w208) -> ()
                n144 = local write "smpl fr*M/N div"(1.0 ("smpl fr*M/N div")) -> ()
                n145 = local write "smpl fr*M/N mul"(1.0 ("smpl fr*M/N mul")) -> ()
              }
              event "btn ok", "btn cancel": Value Change; Panel Close {
                # "Panel Exit"
                n146 = event-data() -> ()  [unwired: 1 in, 3 out]
                n147 = case shown="True" "btn ok" {
                  tunnel: [TRUE w254] -> w229
                  tunnel: [_ w249] -> w228
                  frame False {
                  }
                  frame True {
                    # "build calculation setup"
                    # "do not leave if user canceled file name test"
                    # "build sequence"
                    # "we need sequence\nwth just one item"
                    # "build sampling setup"
                    # "OK pressed - build measurement sequence and store all setup"
                    n148 = local read "session out"() -> (w252:T91)
                    n149 = control-ref of="srate tabs"() -> (w236:refnum<vi>)
                    n150 = Unbundle By Name(w252) -> ("processing setup.QWTB.parsed parameters"=w251:T94[], "processing setup"=w250:T97)
                    n151 = call "Meas Config Panel - Sample Rate Selectors Update.vi"("tab control ref"=w236) -> ("error out"=w235:errorcluster, "sampling rate"=w234:T52)  [unwired: 9 in]
                    n152 = local read "pre-trig ratio"() -> (w233:dbl)
                    n153 = local read "trig coupling"() -> (w273:T4)
                    n154 = call <vilib>:"Clear Errors.vi"("error in (no error)"=w235) -> ()  [unwired: 5 in, 2 out]
                    n155 = local read "trig mode"() -> (w270:T6)
                    n156 = local read "trig slope"() -> (w272:T5)
                    n157 = local read "trig level"() -> (w271:dbl)
                    n158 = local read "trig hyst"() -> (w232:dbl)
                    n159 = local read "range mode"() -> (w267:T3)
                    n160 = local read "smpl count"() -> (w279:i64)
                    n161 = Bundle By Name(cluster=T37 {"source"=enum."Immediate", "slope"=enum."POS", "coupling"=enum."DC", "level [V]"=0.0, "hysteresis [V]"=0.0, "pre-trigger [%]"=0.0} ("trigger"), "source"=w270, "level [V]"=w271, "slope"=w272, "coupling"=w273, "hysteresis [V]"=w232, "pre-trigger [%]"=w233) -> (w274:T37)
                    n162 = local read "aperture"() -> (w278:dbl)
                    n163 = call "GUI Update Range Selectors.vi"("range mode"=w267, "odd and even item names"="range odd\nrange even") -> ("ranges vector [V]"=w276:dbl[])  [unwired: 1 in]
                    n164 = Bundle By Name(cluster=T93 {"count [smpl]"=0, "aperture [s]"=0.0, "trigger"={"source"=enum."Immediate", "slope"=enum."POS", "coupling"=enum."DC", "level [V]"=0.0, "hysteresis [V]"=0.0, "pre-trigger [%]"=0.0}, "ranges [Vpk]"=[], "QWTB parameters"=[], "sampling rate"={"freq mode"=enum."fs or Ts", "fs [Hz]"=0.0, "fref [Hz]"=0.0, "mul"=0.0, "div"=0.0}} ("meas config"), "sampling rate"=w234, "count [smpl]"=w279, "aperture [s]"=w278, "ranges [Vpk]"=w276, "trigger"=w274, "QWTB parameters"=w251) -> (w269:T93)
                    n165 = local read "smpl fr*M/N mul"() -> (w240:dbl)
                    n166 = local read "smpl fr*M/N div"() -> (w239:dbl)
                    n167 = local read "smpl fr*M/N fr"() -> (w241:dbl)
                    n168 = local read "smpl abs fr fs"() -> (w244:dbl)
                    n169 = local read "smpl fr*R rat"() -> (w237:dbl)
                    n170 = local read "smpl fr/N div"() -> (w242:dbl)
                    n171 = local read "smpl fr*R fr"() -> (w238:dbl)
                    n172 = local read "range even"() -> (w265:dbl)
                    n173 = local read "meas name"() -> (w262:string)
                    n174 = local read "smpl fr/N fr"() -> (w243:dbl)
                    n175 = local read "data folder"() -> (w263:path)
                    n176 = local read "smpl abs fr"() -> (w245:dbl)
                    n177 = local read "avg cycles"() -> (w246:i32)
                    n178 = local read "range odd"() -> (w264:dbl)
                    n179 = local read "rec cycles"() -> (w260:i32)
                    n180 = local read "rec delay"() -> (w248:dbl)
                    n181 = local read "comment"() -> (w247:string)
                    n182 = local read "fs mode"() -> (w266:T2)
                    n183 = local read "meas id"() -> (w253:i32)
                    n184 = Build Array(w269) -> (w261:T93[])
                    n185 = Bundle By Name(cluster=T95 {"group setups"=[], "rec count"=0, "range mode"=enum."Keep defaults", "fs mode"=enum."Frequency", "rng even"=0.0, "rng odd"=0.0, "folder"=path "", "name base"="", "meas id"=0, "settle [s]"=0.0, "comment"="", "avg count"=0, "fs-abs-fr fr"=0.0, "fs-abs-fr fs"=0.0, "fs-div fr"=0.0, "fs-div div"=0.0, "fs-mn fr"=0.0, "fs-mn mul"=0.0, "fs-mn div"=0.0, "fs-rat fr"=0.0, "fs-rat rat"=0.0} ("sequence setup"), "group setups"=w261, "rec count"=w260, "range mode"=w267, "fs mode"=w266, "rng even"=w265, "rng odd"=w264, "folder"=w263, "name base"=w262, "meas id"=w253, "settle [s]"=w248, "comment"=w247, "avg count"=w246, "fs-abs-fr fr"=w245, "fs-abs-fr fs"=w244, "fs-div fr"=w243, "fs-div div"=w242, "fs-mn fr"=w241, "fs-mn mul"=w240, "fs-mn div"=w239, "fs-rat fr"=w238, "fs-rat rat"=w237) -> (w257:T95)
                    n186 = call "Meas Generate Sequence.vi"("processing setup"=w250, "sequence setup"=w257) -> ("error out"=w259:errorcluster, "sequence out"=w258:T92[])  [unwired: 7 in, 1 out]
                    n187 = call "Meas Check Sequence Files.vi"("error in"=w259, "sequence setup"=w257) -> ("error out"=w249:errorcluster, "cancel?"=w255:bool, "sequence setup out (copy)"=w256:T95)  [unwired: 7 in]
                    n188 = case shown="False" w255 {
                      tunnel: w258 -> [w283 _]
                      tunnel: w256 -> [w282 _]
                      frame False {
                        # "update session with new setup"
                        n189 = local read "calc result?"() -> (w281:bool)
                        n190 = local read "session out"() -> (w285:T91)
                        n191 = Bundle By Name(cluster=w285, "processing setup.calculate?"=w281, "sequence"=w283, "sequence setup"=w282) -> (w284:T91)
                        n192 = local write "session out"(w284) -> ()
                      }
                      frame True {
                      }
                    }
                    n193 = Not(x=w255) -> (.not. x?=w254:bool)
                  }
                }
              }
              event "btn proc": Value Change {
                # "DATA PROCESSING SETUP"
                n194 = event-data() -> ()  [unwired: 1 in, 6 out]
                n195 = local read "session out"() -> (w288:T91)
                n196 = call "Meas Process Config Panel.vi"("session in"=w288) -> ("error out"=w286:errorcluster, "session out"=w287:T91)  [unwired: 9 in]
                n197 = local write "session out"(w287) -> ()
                n198 = call <vilib>:"Clear Errors.vi"("error in (no error)"=w286) -> ()  [unwired: 5 in, 2 out]
              }
              event "smpl time": Value Change {
                n199 = event-data() -> ()  [unwired: 1 in, 6 out]
                n200 = control-ref of="srate tabs"() -> (w292:refnum<vi>)
                n201 = call "Meas Config Panel - Sample Rate Selectors Update.vi"("tab control ref"=w292) -> ("error out"=w291:errorcluster, "sampling rate"=w290:T52)  [unwired: 9 in]
                n202 = local read "smpl time"() -> (w295:dbl)
                n203 = call <vilib>:"Clear Errors.vi"("error in (no error)"=w291) -> ()  [unwired: 5 in, 2 out]
                n204 = Unbundle By Name(w290) -> ("fs [Hz]"=w289:dbl)
                n205 = Multiply(x=w295, y=w289) -> (x*y=w294:dbl)
                n206 = To Quad Integer(1:w294) -> (0:w293:i64)
                n207 = local write "smpl count"(w293) -> ()
              }
              event "smpl count": Value Change {
                n208 = event-data() -> ()  [unwired: 1 in, 6 out]
                n209 = control-ref of="srate tabs"() -> (w299:refnum<vi>)
                n210 = local read "smpl count"() -> (w302:i64)
                n211 = call "Meas Config Panel - Sample Rate Selectors Update.vi"("tab control ref"=w299) -> ("error out"=w298:errorcluster, "sampling rate"=w297:T52)  [unwired: 9 in]
                n212 = Unbundle By Name(w297) -> ("fs [Hz]"=w296:dbl)
                n213 = To Double Precision Float(number=w302) -> (double precision float=w301:dbl)
                n214 = call <vilib>:"Clear Errors.vi"("error in (no error)"=w298) -> ()  [unwired: 5 in, 2 out]
                n215 = Divide(x=w301, y=w296) -> (x/y=w300:dbl)
                n216 = local write "smpl time"(w300) -> ()
              }
              event "smpl rate", "smpl abs fr", "smpl abs fr fs", "smpl fr/N fr", "smpl fr/N div", "smpl fr/N fs", "smpl fr*M/N fr", "smpl fr*M/N div", "smpl fr*M/N fs", "smpl fr*M/N mul", "smpl fr*R fr", "smpl fr*R rat", "smpl fr*R fs": Value Change {
                # "query ADC capabilities"
                n217 = event-data() -> ("CtlRef"=w318:refnum<vi>)  [unwired: 1 in, 5 out]
                n218 = control-ref of="fs mode"() -> (w317:refnum<vi>)
                n219 = Equal?(x=w317, y=w318) -> (x = y?=w316:bool)
                n220 = case shown="True" w316 {
                  tunnel: [_ w323] -> w315
                  frame False {
                  }
                  frame True {
                    n221 = property on="smpl rate" class="DigNum (strict)"() -> (error out=w324:errorcluster, "Value"=w326:dbl)  [unwired: 2 in, 1 out]
                    n222 = Reciprocal(x=w326) -> (1/x=w325:dbl)
                    n223 = property on="smpl rate" class="DigNum (strict)"(error in=w324, "Val(Sgnl)"=w325) -> (error out=w323:errorcluster)  [unwired: 1 in, 1 out]
                  }
                }
                n224 = control-ref of="srate tabs"() -> (w306:refnum<vi>)
                n225 = call "Meas Config Panel - Sample Rate Selectors Update.vi"("error in (no error)"=w315, "tab control ref"=w306) -> ("error out"=w310:errorcluster, "sampling rate"=w322:T52)  [unwired: 8 in]
                n226 = local read "aperture"() -> (w312:dbl)
                n227 = Unbundle By Name(w322) -> ("fs [Hz]"=w309:dbl)
                n228 = Bundle By Name(cluster=T113 {"fs [Hz]"=0.0, "aperture [s]"=0.0} ("parameters"), "fs [Hz]"=w309, "aperture [s]"=w312) -> (w313:T113)
                n229 = local read "adc"() -> (w314:T7)
                n230 = call "ADC Get Capabilities.vi"("error in"=w310, "parameters"=w313, "adc session in"=w314) -> ("error out"=w308:errorcluster, "capabilities"=w307:T115)  [unwired: 6 in, 1 out]
                n231 = call "Meas Config Panel - Sample Rate Selectors Update.vi"("error in (no error)"=w308, "adc capabilities"=w307, "tab control ref"=w306) -> ("error out"=w305:errorcluster, "sampling rate"=w304:T52)  [unwired: 7 in]
                n232 = local read "smpl time"() -> (w321:dbl)
                n233 = Unbundle By Name(w304) -> ("fs [Hz]"=w303:dbl)
                n234 = call <vilib>:"Clear Errors.vi"("error in (no error)"=w305) -> ()  [unwired: 5 in, 2 out]
                n235 = Multiply(x=w321, y=w303) -> (x*y=w320:dbl)
                n236 = To Quad Integer(1:w320) -> (0:w319:i64)
                n237 = local write "smpl count"(w319) -> ()
              }
              event "btn assist": Value Change {
                # "initiate coherent setup finder assistant"
                n238 = event-data() -> ()  [unwired: 1 in, 6 out]
                n239 = local read "fs mode"() -> (w333:T2)
                n240 = control-ref of="srate tabs"() -> (w331:refnum<vi>)
                n241 = call "Meas Config Panel - Sample Rate Selectors Update.vi"("tab control ref"=w331) -> ("error out"=w330:errorcluster, "sampling rate"=w329:T52)  [unwired: 9 in]
                n242 = local read "session out"() -> (w336:T91)
                n243 = Unbundle By Name(w329) -> ("fs [Hz]"=w327:dbl)
                n244 = call <vilib>:"Clear Errors.vi"("error in (no error)"=w330) -> ("error out"=w328:errorcluster)  [unwired: 5 in, 1 out]
                n245 = call "Assist Sampling Setup Panel.vi"("error in"=w328, "fs in [Hz]"=w327, "session in"=w336) -> ("error out"=w337:errorcluster, "ok"=w332:bool, "smpl setup"=w334:T117, "session out"=w335:T91)  [unwired: 5 in]
                n246 = local write "session out"(w335) -> ()
                n247 = call <vilib>:"Clear Errors.vi"("error in (no error)"=w337) -> ()  [unwired: 5 in, 2 out]
                n248 = case shown="True" w332 {
                  tunnel: w334 -> [_ w341]
                  tunnel: w333 -> [_ w340]
                  frame False {
                  }
                  frame True {
                    n249 = Unbundle By Name(w341) -> ("N"=w338:i64, "fs [Hz]"=w339:ext)
                    n250 = case shown="\"Period\"" w340 {
                      tunnel: w339 -> [w342 w344]
                      frame "Frequency", Default {
                        n251 = local write "smpl rate"(w342) -> ()
                      }
                      frame "Period" {
                        n252 = Reciprocal(x=w344) -> (1/x=w343:ext)
                        n253 = local write "smpl rate"(w343) -> ()
                      }
                    }
                    n254 = local write "smpl count"(w338) -> ()
                  }
                }
              }
            }
          }
        }
        frame Error {
        }
      }
      n255 = Equal?(x=Meas_Sampling_Rate_Mode."Frequency", y=w92) -> (x = y?=w96:bool)
      n256 = Unbundle By Name(w89) -> ("source"=w88:T6, "level [V]"=w87:dbl, "coupling"=w86:T4, "slope"=w85:T5, "hysteresis [V]"=w28:dbl, "pre-trigger [%]"=w27:dbl)
      n257 = expression code="max(n,1)"(w50) -> (w29:i64)
      n258 = local write "aperture"(w90) -> ()
      n259 = local write "smpl count"(w29) -> ()
      n260 = To Double Precision Float(number=w29) -> (double precision float=w52:dbl)
      n261 = Reciprocal(x=w95) -> (1/x=w53:dbl)
      n262 = local write "trig mode"(w88) -> ()
      n263 = local write "trig level"(w87) -> ()
      n264 = local write "trig coupling"(w86) -> ()
      n265 = local write "trig slope"(w85) -> ()
      n266 = local write "trig hyst"(w28) -> ()
      n267 = local write "pre-trig ratio"(w27) -> ()
      n268 = Multiply(x=w52, y=w53) -> (x*y=w51:dbl)
      n269 = Select(t=w95, s=w96, f=w53) -> (s? t:f=w91:dbl)
      n270 = local write "smpl time"(w51) -> ()
      n271 = local write "smpl rate"(w91) -> ()
      n272 = Not(x=w99) -> (.not. x?=w55:bool)
      n273 = Merge Errors(w49, w48) -> (w47:errorcluster)
      n274 = flat-sequence {
        tunnel: w55 -> [_]
        tunnel: w46 -> [w106]
        frame #0 {
          # "on exit action"
          n275 = call "SGUI Register Controls.vi"("register mode (overwrite)"=SGUI_Assign_References_Mode."Release ID", "controls ID (empty)"=w106) -> ("error out"=w111:errorcluster)  [unwired: 15 in, 2 out]
          n276 = call <vilib>:"Clear Errors.vi"("error in (no error)"=w111) -> ("error out"=w108:errorcluster)  [unwired: 5 in, 1 out]
          n277 = Current VI's Path() -> (path=w110:path)
          n278 = call "GUI Panel Control.vi"("action (open panel)"=GUI_Panel_Control_Action."Close panel", "error in (no error)"=w108, "vi path"=w110) -> ("error out"=w107:errorcluster)  [unwired: 8 in]
          n279 = call <vilib>:"Clear Errors.vi"("error in (no error)"=w107) -> ()  [unwired: 5 in, 2 out]
        }
      }
    }
  }
  "canceled?" <- w4
  "error out" <- w3
  "session out" <- "session in"
